vi "DAISY_PAR_HV_slow_control_2_16.vi"() -> ()   [LabVIEW 2018]
uses:
  4623b864-5764-45c6-9cb2-3e18237880ca.vi
  fa57f61f-0bb9-49ac-92eb-fcb40add4dbb.vi
  <vilib>/DAQmx/read.llb/DAQmx Read (Analog 1D DBL NChan 1Samp).vi
  ffb0d1b3-ef19-4e2e-b36e-7277177ef4b3.vi
  9a1acc8a-69db-4048-9e4c-bb07d66d2422.vi
  <vilib>/DAQmx/create/channels.llb/DAQmx Create Channel (AI-Voltage-Basic).vi
  <vilib>/DAQmx/create/channels.llb/DAQmx Create Channel (AI-Current-Basic).vi
  <vilib>/DAQmx/create/channels.llb/DAQmx Create Channel (AI-Temperature-RTD).vi
  <vilib>/DAQmx/miscellaneous.llb/DAQmx Fill In Error Info.vi
  <vilib>/Utility/file.llb/Read Delimited Spreadsheet (string).vi
  <instrlib>/Lake Shore 335/Lake Shore 335.lvlib
  <instrlib>/CAEN PSM/CAEN PSM.lvlib
  <resource>/objmgr/daqmx.rc
panel:
  out "Setpoint (°C)":dbl
  out "Heater Range":i32
  out "Heater (°C)":dbl
  out "Coldhead (°C)":dbl
  out "Cycle number":i32
  out "Alarm state":bool
  out "Timestamp last \nmeasured (UPS)":timestamp
  out "Auto-clear":bool
  in  "Auto-clear data?":bool
  in  "Clear data":bool
  in  "Clear data every N cycles":dbl=1000000.0
  in  "N samples":i32=30
  out "Average Flow (SLPM)":dbl caption="Flow (SLPM)"
  out "CAEN Ch. Names":string[](array[string])
  in  "Cycles to execute":dbl=5.0 format="%#_13g"
  out "Detector Pressure":dbl
  in  "N samples":i32=20
  in  "Allows tabs on \nfront panel":T1(tab)
  in  "Anode ch.":enum16{"1", "2", "3", "4"}(ring)=enum."3"
  in  "CAEN unit selector":enum16{"CAEN 1", "CAEN 2"}(ring)
  in  "Multipliers":dbl[](array[numeric])=[1.0, 1.0, 1.0, 1.0, 1.0, 1.0, 1.0, 1.0]
  in  "Offsets\nsubtracted":dbl[](array[numeric])=[0.0, 0.0, 0.0, 0.0, 0.0, 0.0, 0.0, 0.0]
  in  "Channel Names (9207, ai8:15)":string[](array[string])=["i0", "i1", "i2", "i3", "i4", "i5", "i6", "i7"] caption="\"Other\""
  in  "Flow meter input:":u16(ring)=3 items=["v0", "v1", "v2", "v3", "v4", "v5", "v6", "v7"]
  in  "Detector pressure input:":u16(ring) items=["v0", "v1", "v2", "v3", "v4", "v5", "v6", "v7"]
  in  "Channel Names (9207, ai0:7)":string[](array[string])=["v0", "v1", "v2", "v3", "v4", "v5", "v6", "v7"] caption="\"Other\""
  in  "Multipliers":dbl[](array[numeric])=[1.0, 1.0, 1.0, 1.0, 1.0, 1.0, 1.0, 1.0]
  in  "Offsets\nsubtracted":dbl[](array[numeric])=[0.0, 0.0, 0.0, 0.0, 0.0, 0.0, 0.0, 0.0]
  in  "Voltage channels":tag[](array[tag])=["9207/ai0", "9207/ai1", "9207/ai2", "9207/ai3", "9207/ai4", "9207/ai5", "9207/ai6", "9207/ai7"]
  in  "COM-port CAEN":refnum<visa-resource-name>
  in  "ID Query":bool
  in  "COM-port LakeShore":refnum<visa-resource-name>
  in  "PID settings":cluster{"P":dbl, "I":dbl, "D":dbl}={"P"=50.0, "I"=20.0, "D"=120.0}
  in  "Current channels":tag[](array[tag])=["9207/ai8", "9207/ai9", "9207/ai10", "9207/ai11", "9207/ai12", "9207/ai13", "9207/ai14", "9207/ai15"]
  in  "Channel Names (CAEN)":string[](array[string])=["PMT 1", "PMT 2", "Anode", "Cathode", "Top gate", "Bottom gate", "Other 1", "Other 2"]
  in  "RTD Type":i32(ring)=10071 items=["Pt3750"=12481, "Pt3851"=10071, "Pt3911"=12482, "Pt3916"=10069, "Pt3920"=10053, "Pt3928"=12483, "Custom"=10137]
  in  "Module 1 channels (slot 1)":tag[](array[tag])=["cDAQ2Mod2/ai0", "cDAQ2Mod2/ai1", "cDAQ2Mod2/ai2", "cDAQ2Mod2/ai3", "cDAQ2Mod2/ai4", "cDAQ2Mod2/ai5", "cDAQ2Mod2/ai6", "cDAQ2Mod2/ai7"]
  in  "Resistance Configuration":i32(ring)=3 items=["3-Wire"=3, "4-Wire"=4]
  in  "R (T = 0°C):":dbl=100.0 format="%_4g"
  in  "B":dbl
  in  "A":dbl
  in  "C":dbl
  in  "Module 2 channels (slot 2)":tag[](array[tag])=["cDAQ2Mod3/ai0", "cDAQ2Mod3/ai1", "cDAQ2Mod3/ai2", "cDAQ2Mod3/ai3", "cDAQ2Mod3/ai4", "cDAQ2Mod3/ai5", "cDAQ2Mod3/ai6", "cDAQ2Mod3/ai7"]
  in  "Shut off heater \nif Alarm is active":bool=TRUE
  in  "Re-save headers":bool
  in  "Resistance Configuration":i32(ring)=3 items=["3-Wire"=3, "4-Wire"=4]
  in  "Module 3 channels":tag[](array[tag])
  in  "RTD Type":i32(ring)=12481 items=["Pt3750"=12481, "Pt3851"=10071, "Pt3911"=12482, "Pt3916"=10069, "Pt3920"=10053, "Pt3928"=12483, "Custom"=10137]
  in  "R (T = 0°C)":dbl=1000.0 format="%0.1f"
  in  "Ignore Initialization Errors":bool=TRUE caption="Ignore init. errors?"
  out "Started up?":bool
  in  "9216 Timing Mode":i32(ring)=14712 items=["High Resolution"=10195, "High Speed"=14712]
  in  "9207 Timing Mode":i32(ring)=14712 items=["High Resolution"=10195, "High Speed"=14712]
  in  "9226 Timing Mode":i32(ring)=14712 items=["High Resolution"=10195, "High Speed"=14712]
  in  "Kill all channels (Trip)":bool
  in  "Scale.Range:Minimum 8":dbl
  in  "Scale.Range:Maximum 8":dbl=4000.0
  in  "Scale.Range:Minimum 7":dbl
  in  "Scale.Range:Maximum 7":dbl=4000.0
  in  "Scale.Range:Minimum 6":dbl=-3000.0
  in  "Scale.Range:Maximum 6":dbl
  in  "Scale.Range:Minimum 5":dbl
  in  "Scale.Range:Maximum 5":dbl=3000.0
  in  "Scale.Range:Minimum 4":dbl=-5000.0
  in  "Scale.Range:Maximum 4":dbl
  in  "Scale.Range:Maximum 3":dbl=4000.0
  in  "Scale.Range:Minimum 3":dbl
  in  "Scale.Range:Maximum 2":dbl=1000.0
  in  "Scale.Range:Minimum 2":dbl
  out "CAEN 1.1":dbl(knob) scale=0.0..1000.0
  out "CAEN 1.1":string
  in  "Scale.Range:Maximum":dbl=1000.0
  in  "Scale.Range:Minimum":dbl
  out "CAEN 2.3 2":string
  out "CAEN 2.2 2":string
  out "Channel Names":string[](array[string])
  out "CAEN 2.3":dbl(knob) scale=0.0..4000.0
  out "CAEN 2.2":dbl(knob) scale=0.0..4000.0
  out "CAEN 2.1":string
  out "CAEN 2.0":string
  out "CAEN 1.3":string
  out "CAEN 1.2":string
  out "CAEN 1.0":string
  out "Channel Names":string[](array[string])
  in  "Set to zero (ramp down)":bool
  out "CAEN 2.1":dbl(knob) scale=0.0..-3000.0
  out "CAEN 2.0":dbl(knob) scale=0.0..3000.0
  in  "Apply Voltage":bool
  in  "VSet (V)":dbl[](array[numeric])
  in  "IMax (uA)":sgl[](array[numeric])
  in  "VMax (V)":u16[](array[numeric])
  out "CAEN 1.3":dbl(knob) scale=0.0..-5000.0
  out "CAEN 1.2":dbl(knob) scale=0.0..4000.0
  out "CAEN 1.0":dbl(knob) scale=0.0..1000.0
  out "Vmon (V)":dbl[](array[numeric])
  out "IMon (uA)":dbl[](array[numeric])
  in  "Reset anode\nperiodically?":bool
  in  "Kill every Y minutes":i32=10
  in  "Keep off for X seconds":i32=10
  out "?":bool
  out "Killed":bool
  out "Restarted":bool
  out "Anode timers":timestamp[](array[timestamp])
  out "Seconds until \nanode autokill":dbl format="%.2g"
  out "Seconds until \nanode reset":dbl format="%.2g"
  in  "Temperature channel selector":u16(ring) items=["0"=0, "1"=1, "2"=2, "3"=3, "4"=4, "5"=5, "6"=6, "7"=7, "Average"=666]
  out "Heater power (%)":cluster{timestamp[], dbl[]}[](graph)
  out "Flow (SLPM)":cluster{timestamp[], dbl[]}[](graph)
  out "9207 (ai 0:7, Volts)":cluster{timestamp[], dbl[]}[](graph)
  out "Phase Diagram":cluster{"X":dbl, "Y":dbl}[](graph)
  out "Setup Temperature (9216 0:15, °C)":cluster{timestamp[], dbl[]}[](graph)
  out "LakeShore readings":dbl[](array[numeric])
  out "Low Temperature (9226 0:7 and LakeShore A;B, °C)":cluster{timestamp[], dbl[]}[](graph)
  in  "Reset?":bool
  out "Integrated Flow (SL)":dbl
  in  "Pause?":bool
  in  "Setpoint (°C)":dbl=-100.0 format="%.1f"
  in  "Heater range":u16(ring) items=["Off", "Low (On)", "Medium", "High"]
  in  "\"Sound\" alarm":bool
  in  "Sound alarm\nFrequency (Hz)":dbl=1260.0
  in  "Send status email now":bool
  out "Email error":i32
  out "source":string
  in  "Number of Bonus lines":i32=1
  out "Names (optional)":string[](array[string])
  in  "Send daily email?":bool=TRUE
  in  "Phone numbers":string[](array[string])
  out "Alarm (or test) message":string
  in  "Alarm\nMaster switch":bool
  in  "Repeat Alarm SMS\nevery N minutes":dbl=15.0
  in  "Test alarm":bool
  out "Warning":bool
  in  "UPS":bool
  in  "UPS Voltage \nLower Threshold":dbl=220.0
  out "NI mod 2&3 status":bool
  in  "NI mod 2&3":bool
  in  "NI mod 1":bool
  in  "CAEN 2":bool
  in  "CAEN 1":bool
  in  "LakeShore":bool
  out "Det. P. warning":bool
  out "Boolean 6":bool
  out "Boolean 5":bool
  out "Boolean 4":bool
  out "Boolean 3":bool
  out "Boolean 2":bool
  out "Boolean":bool
  in  "T 6":bool
  in  "T 5":bool
  in  "T 4":bool
  in  "T 3":bool
  in  "T 2":bool
  in  "T 1":bool
  in  "Detector Pressure":bool
  in  "Overpressure threshold":dbl
  in  "Underpressure threshold":dbl
  out "Comm. status":bool
  in  "High Temp threshold":dbl format="%#_13g"
  in  "Low Temp threshold":dbl format="%#_13g"
  out "LakeShore status":bool
  out "NI mod1 (P) status":bool
  out "CAEN 1 status":bool
  out "CAEN 2 status":bool
  out "Initialization status":bool
  out "Minimum input voltage measured":dbl
  out "Alarm active 2":bool
  out "SMS error":string
  out "Status email preview":string
  in  "Send status email at time:":string="14:00"
  in  "Email Addresses":string[](array[string])
  in  "return address":string="xamsups@gmail.com"
  out "NI 9226":errorcluster
  in  "HV Channel status":string="Click the button to request the latest High Voltage channel status.\nView another channel with the arrows, or typing 0 through 3."
  out "CAEN 1":T2(array[cluster])
  out "CAEN 2":T2(array[cluster])
  in  "Query HV status":bool
  in  "LabVIEW error code":string="Google this"
  in  "String 7":string="A checkmark means \"No error\" and false. A red X means an error occurred"
  out "\"status\"":bool
  in  "\"source\"":string="This may show two things: the latest executed VI in the task chain, in reverse order, or: which VI produced an error, with a short description. If the error can't easily be resolved, google the code."
  out "NI 9216 x2":errorcluster
  out "CAEN 1":errorcluster
  out "CAEN 2":errorcluster
  out "Lakeshore":errorcluster
  out "NI 9207":errorcluster
  out "Temp A":dbl
  out "Temp B":dbl
  in  "Temperature Channel Selector":u16(ring) items=["0", "1", "2", "3", "4", "5", "6", "7"]
  out "Historical Large Phase Diagram":cluster{dbl[], dbl[]}[](graph)
  out "Large Phase Diagram":cluster{"X":dbl, "Y":dbl}[](graph)
  in  "Temperature Channel Selector":u16(ring) items=["0"=0, "1"=1, "2"=2, "3"=3, "4"=4, "5"=5, "6"=6, "7"=7, "Average"=666]
  out "PT1000 data":dbl[](array[numeric]) format="%0.2f"
  out "9207 (V; A) Converted":dbl[](array[numeric])
  out "9216 #1 (°C)":dbl[](array[numeric])
  out "9216 #2 (°C)":dbl[](array[numeric])
  out "Raw readouts (V, mA)":dbl[](array[numeric]) format="%0.2f"
  out "Det.P input #":i32
  out "Flow input #":i32
  out "PT100 data":dbl[](array[numeric]) format="%0.2f"
  out "Polarity signs":dbl[](array[numeric])
  out "9207 (ai 8:15, Amperes)":cluster{timestamp[], dbl[]}[](graph)
  in  "Kill voltage":bool
  in  "stop":bool
  out "Voltages":dbl[](array[numeric])
  out "Time until next cycle":dbl format="%.3g"
  in  "Time per cycle (s)":i32=2 caption="Time Target (s)"
  # "Moving Averages"
  # "CAEN settings"
  # "NI 9216 Temperature settings"
  # "NI 9207 Voltage settings"
  # "NI 9207 Current settings"
  # "If RTD type is custom,\nspecify the Callendar-\nVan Dusen parameters"
  # "Anode connected to:"
  # "Channel:"
  # "Lakeshore settings"
  # "NI 9226 Temperature settings"
  # "Miscellaneous"
  # "Gain (P) (XX.X)"
  # "Reset (I) (XX.X)"
  # "Rate (D) (X.X%)"
  # "Data"
  # "Scale:"
  # "to"
  # "to"
  # "Scale:"
  # "Time of last reset"
  # "Time of last reactivation"
  # "to"
  # "Scale:"
  # "to"
  # "Scale:"
  # "Settings"
  # "Scale:"
  # "to"
  # "Scale:"
  # "to"
  # "Scale:"
  # "to"
  # "to"
  # "Scale:"
  # "Alarm indicators and arms"
  # "Detector Thresholds"
  # "Daily status email"
  # "SMS and sound alarm"
  # "Alarm conditions"
  # "Temperature channels:"
  # "Uninterruptable Power Supply"
  # "Task/error information"
  # "High Voltage channel status"
  # "Error info example"
  # "Channel"
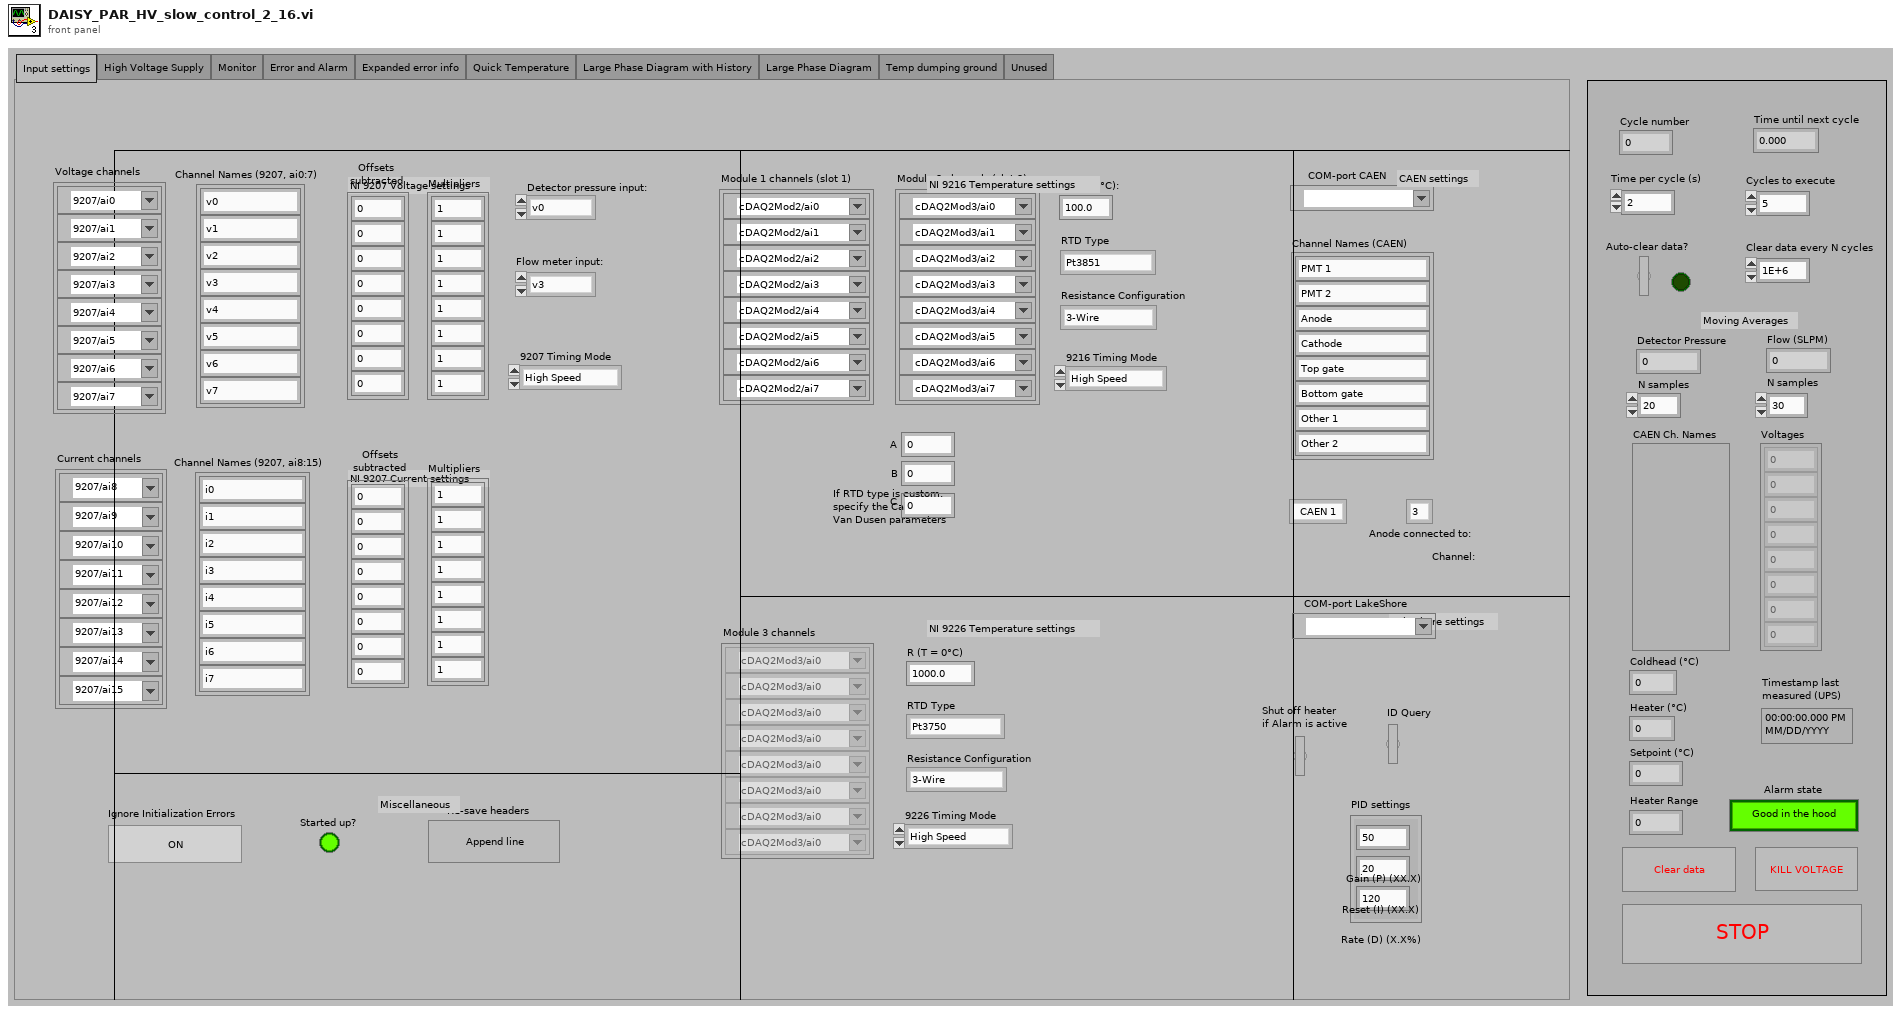
[diagram p1: front panel]
types:
  T1 = enum32{"Input settings", "High Voltage Supply", "Monitor", "Error and Alarm", "Expanded error info", "Quick Temperature", "Large Phase Diagram with History", "Large Phase Diagram", "Temp dumping ground", "Unused"}
  T2 = cluster{"ON":bool, "RUP":bool, "RDW":bool, "OVC":bool, "OVV":bool, "UNV":bool, "MAXV":bool, "TRIP":bool, "OVP":bool, "OVT":bool, "DIS":bool, "KILL":bool, "ILK":bool, "NOCAL":bool}[]
  T3 = cluster{"Baud Rate":u32, "Parity":u16, "Data Bits":u16, "Stop Bits":u16, "Flow Control":u16}
  T4 = typedef "CAEN PSM.lvlib/BoardHandle.ctl" = cluster{"VISA resource name":refnum<visa-resource-name>, "Board address":u8, "NChannels":u8}
  T5 = cluster{"task out":refnum<k21>, "error out":errorcluster}
  T6 = cluster{"VISA resource name out":refnum<visa-resource-name>, "error out":errorcluster}
  T7 = cluster{"VISA resource name":refnum<visa-resource-name>, "Board address":u8, "NChannels":u8}[]
  T8 = cluster{"VISA resource name":refnum<visa-resource-name>, "Board address":u8, "NChannels":u8}
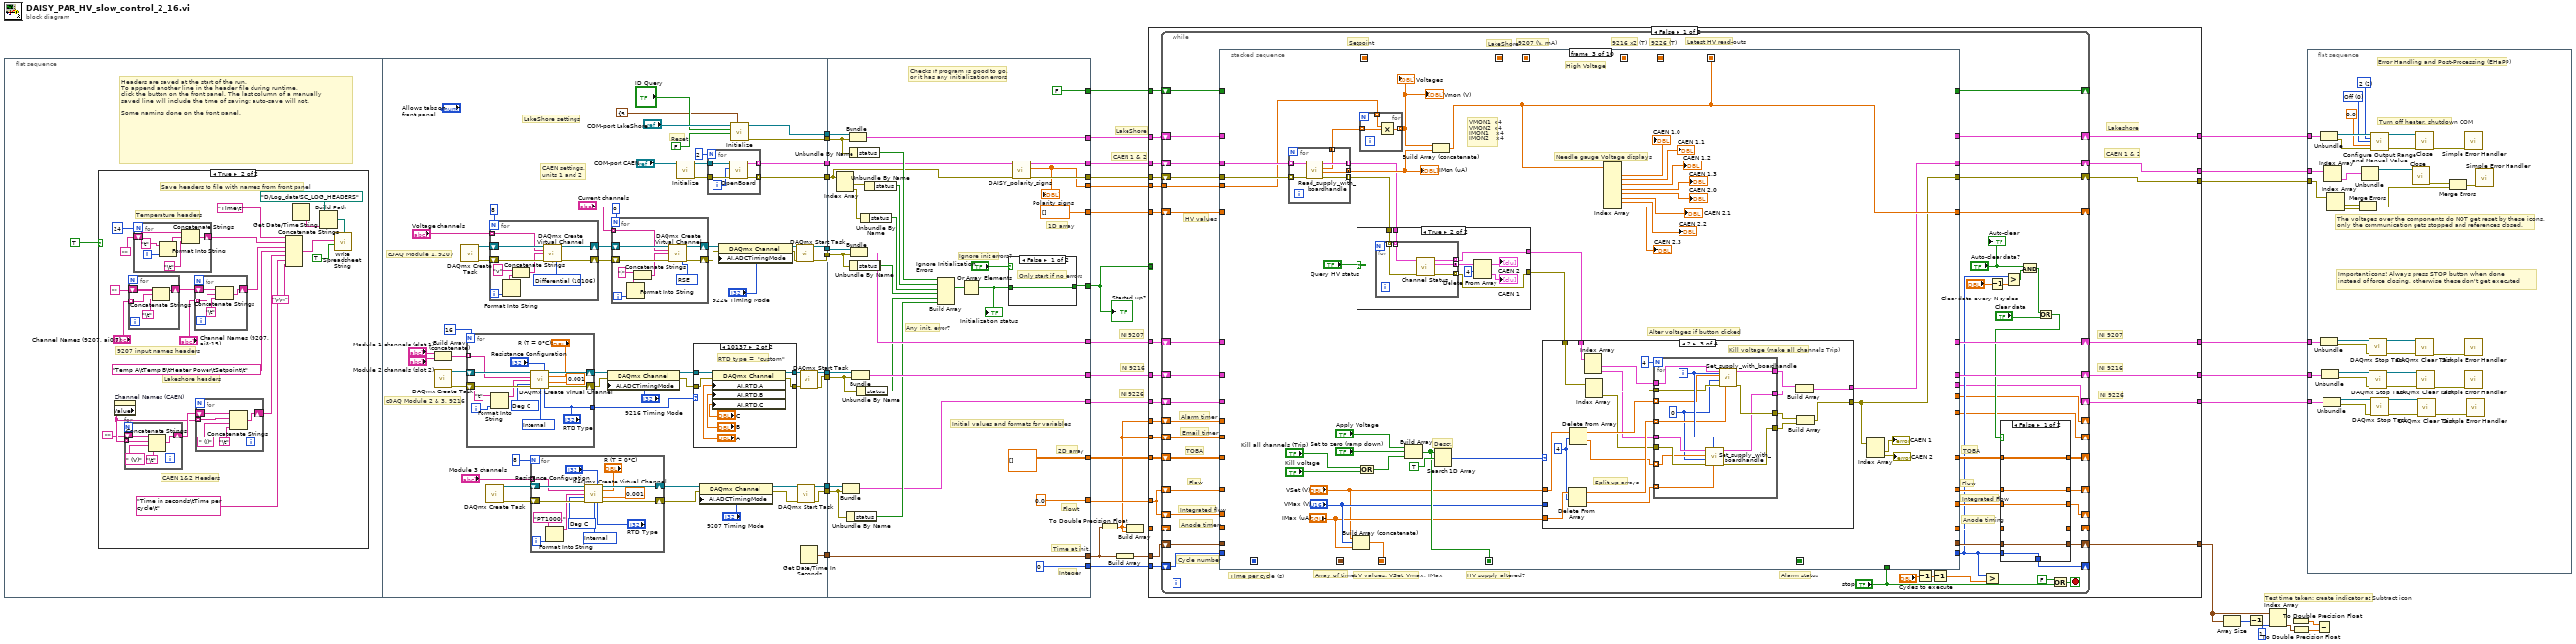
[diagram p0: block diagram]
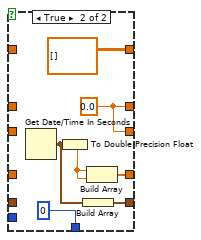
[diagram p2: hidden frame]
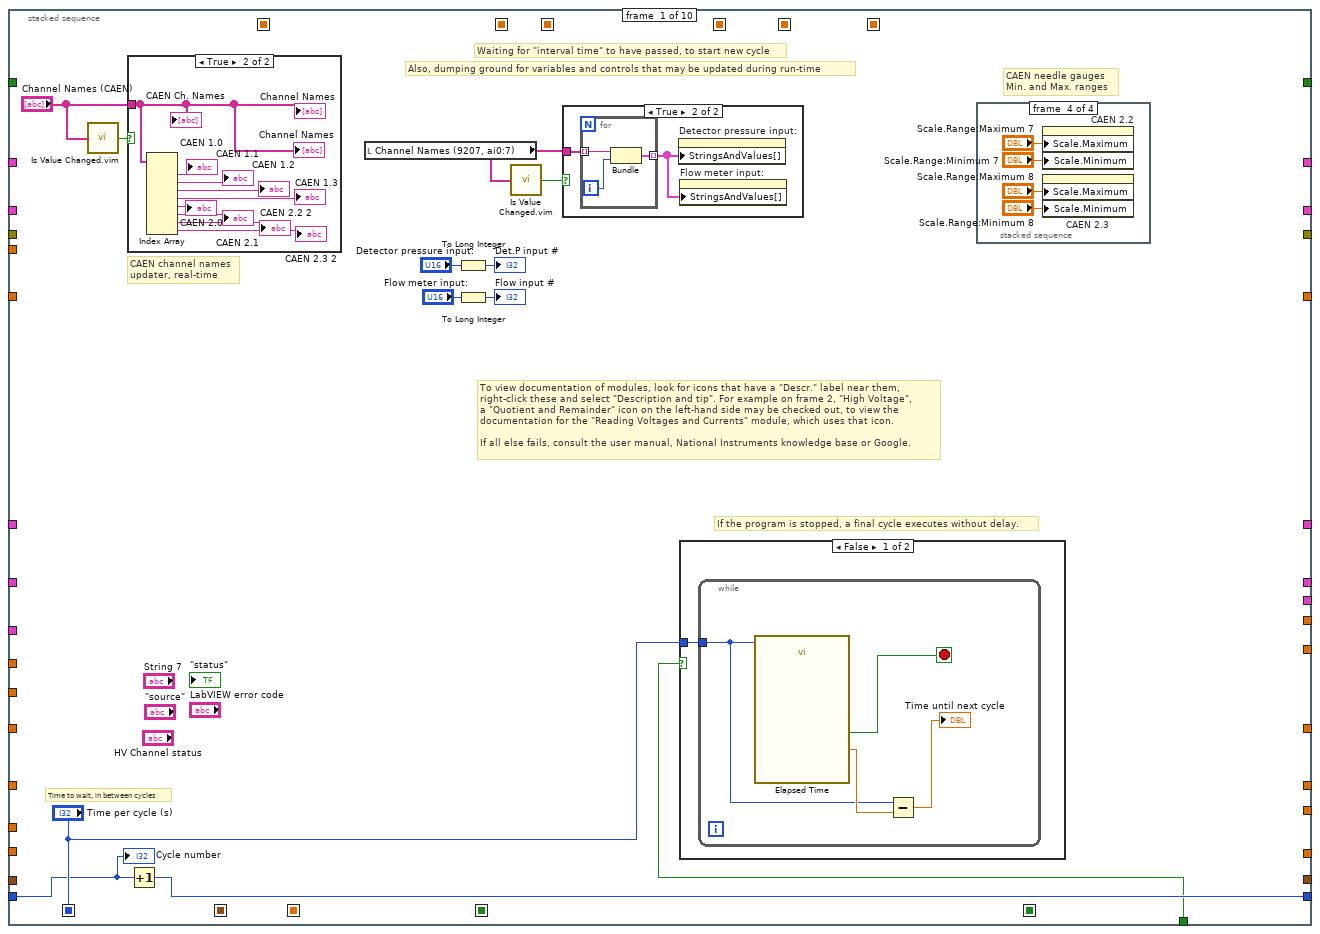
[diagram p3: hidden frame]
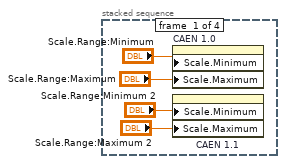
[diagram p6: hidden frame]
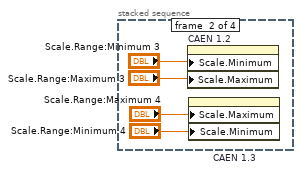
[diagram p7: hidden frame]
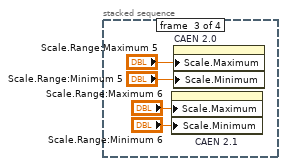
[diagram p8: hidden frame]
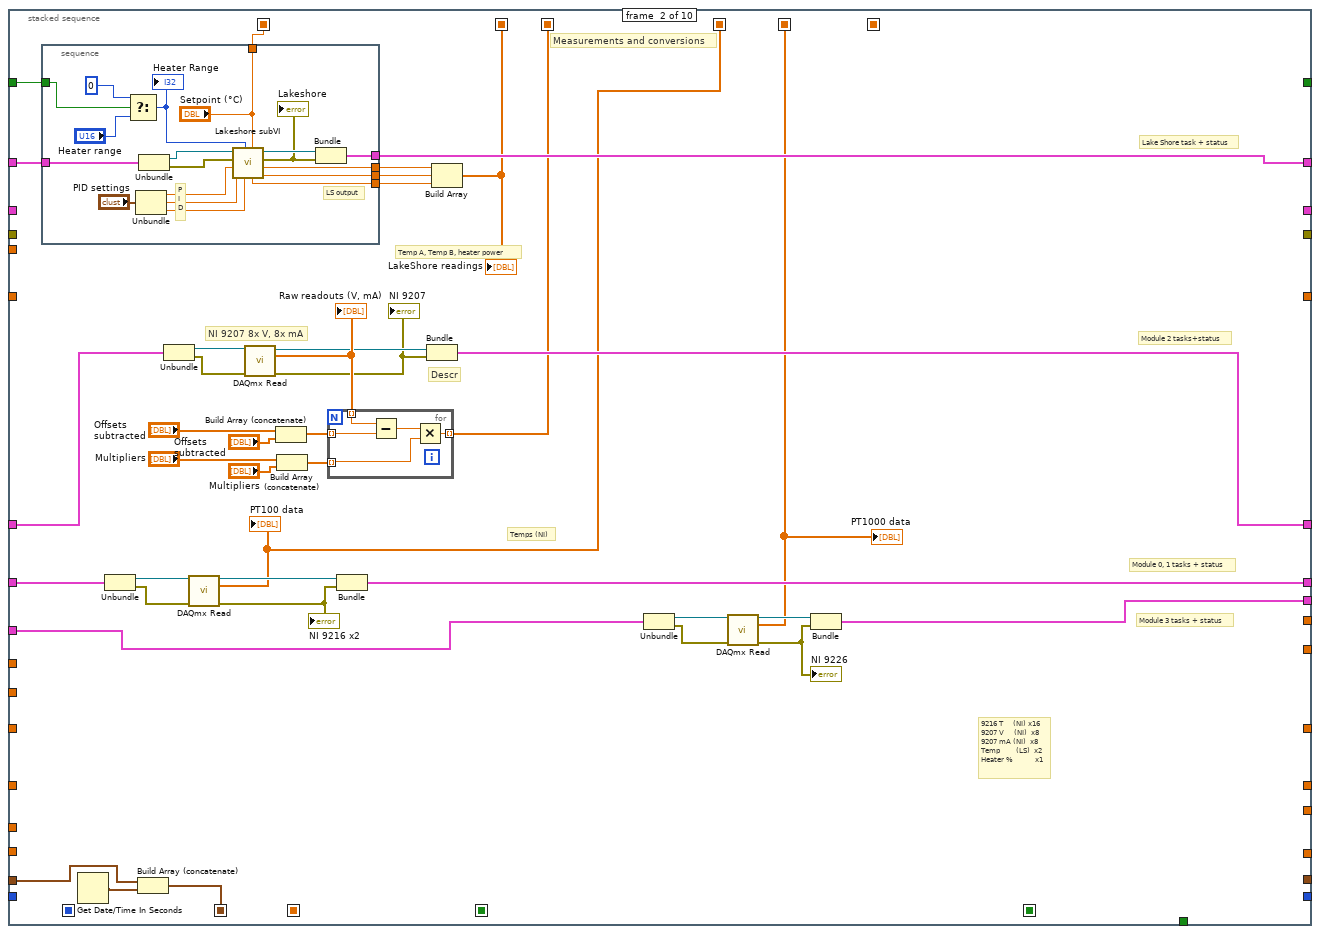
[diagram p10: hidden frame]
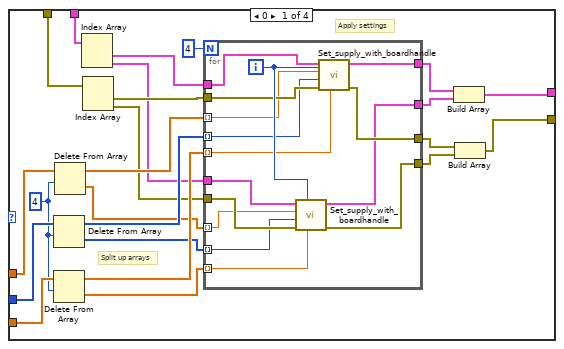
[diagram p11: hidden frame]
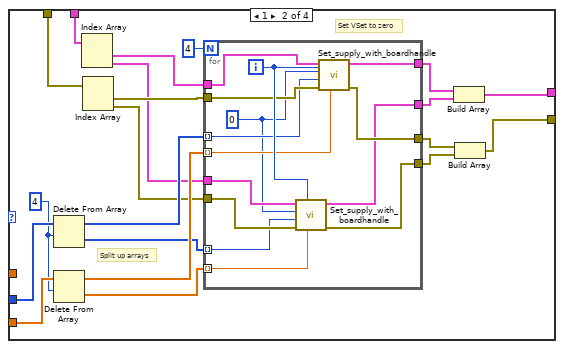
[diagram p12: hidden frame]
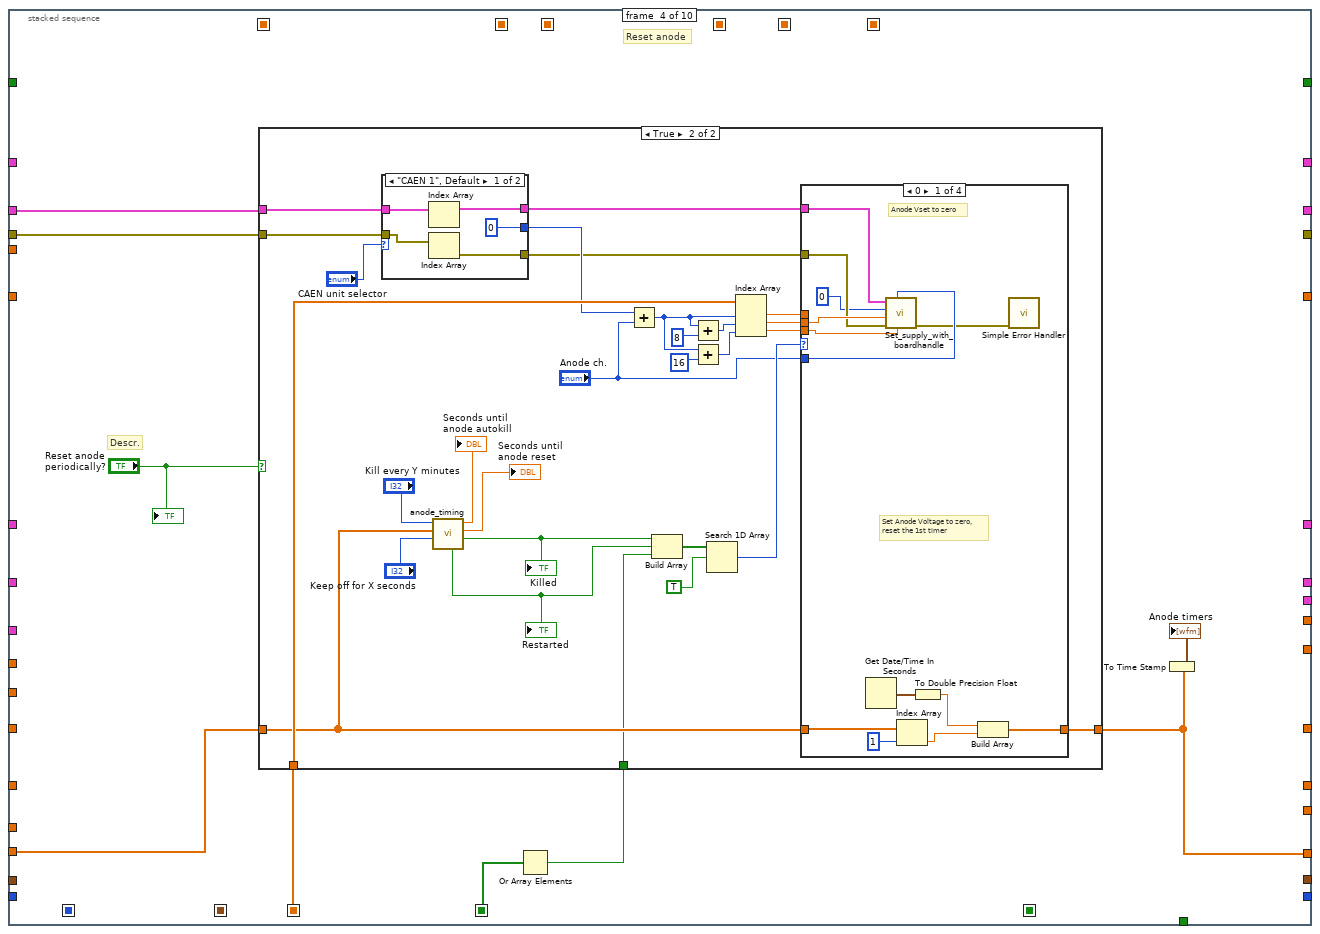
[diagram p15: hidden frame]
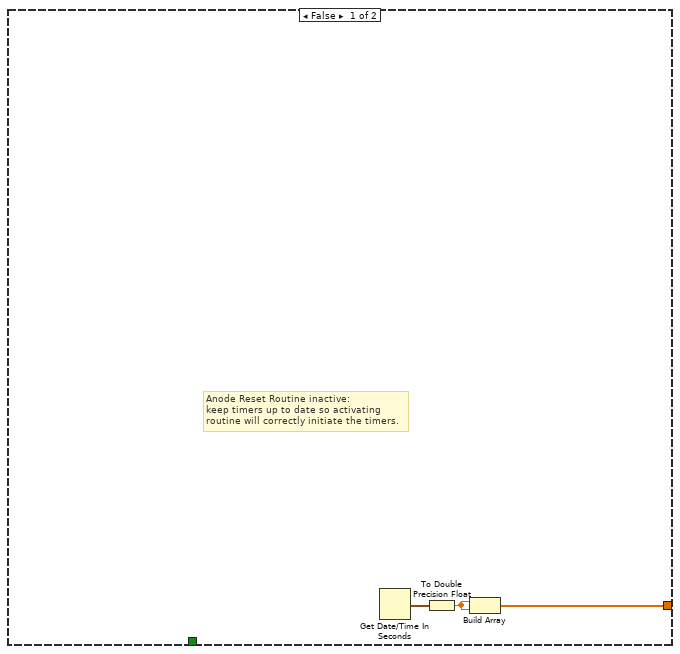
[diagram p16: hidden frame]
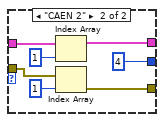
[diagram p17: hidden frame]
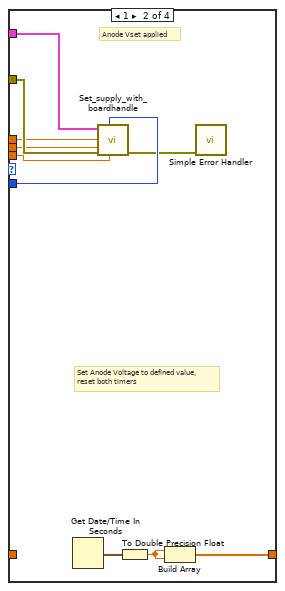
[diagram p18: hidden frame]
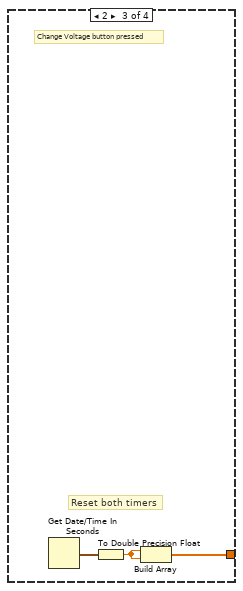
[diagram p19: hidden frame]
diagram:
  # "NI 9226"
  # "NI 9216"
  # "Test time taken: create indicator at Subtract icon"
  # "NI 9207"
  # "CAEN 1 & 2"
  # "LakeShore"
  n1 = flat-sequence {
    tunnel: [w140] -> w42
    tunnel: [w139] -> w41
    tunnel: [w136] -> w40
    tunnel: [w127] -> w39
    tunnel: [w135] -> w35
    tunnel: [w128] -> w21
    tunnel: [w122] -> w14
    tunnel: [w121] -> w13
    tunnel: [w110] -> w9
    tunnel: [w109] -> w8
    tunnel: [w106] -> w4
    tunnel: w42 -> [w237]
    tunnel: w41 -> [w236]
    tunnel: w40 -> [w208]
    tunnel: w39 -> [w229]
    tunnel: [w238] -> w27
    tunnel: [0.0] -> w26
    tunnel: [dbl[] []] -> w38
    tunnel: [dbl[][] []] -> w15
    tunnel: [0] -> w37
    tunnel: [w235] -> w36
    tunnel: [w234] -> w25
    tunnel: w35 -> [w234]
    tunnel: [FALSE] -> w22
    tunnel: w21 -> [w230]
    tunnel: [w228] -> w20
    tunnel: w14 -> [w221]
    tunnel: w13 -> [w220]
    tunnel: [w219] -> w12
    tunnel: w9 -> [w216]
    tunnel: w8 -> [w215]
    tunnel: [w213] -> w7
    tunnel: [w206] -> w5
    tunnel: w4 -> [w210]
    tunnel: [w209] -> w3
    tunnel: [w207] -> w2
    frame #0 {
      # "Headers are saved at the start of the run.\nTo append another line in the header file during runtime,\nclick the button on the front panel. The last column of a manually\nsaved line will include the time of saving; auto-save will not.\n\nSome naming done on the front panel."
      n2 = case shown="True" TRUE {
        frame False {
        }
        frame True {
          # "CAEN 1&2 Headers"
          # "Lakeshore headers"
          # "9207 input names headers"
          # "Temperature headers"
          # "Save headers to file with names from front panel"
          n3 = property on="Channel Names (CAEN)" class="Arr (strict)"() -> ("Value"=w49:string[])  [unwired: 2 in, 2 out]
          n4 = for {
            tunnel: w49 -> [w73] mode=indexing
            shift-right: [w71] -> w50
            shift-left: "" -> [w70]
            n5 = Concatenate Strings(w70, w73, " (V)", "\t") -> (w71:string)
          }
          n6 = for {
            shift-right: [w81] -> w53
            shift-left: "" -> [w82]
            tunnel: "Channel Names (9207, ai0:7)" -> [w79] mode=indexing
            n7 = Concatenate Strings(w82, w79, "\t") -> (w81:string)
          }
          n8 = for {
            N: 24 -> [_]
            shift-right: [w83] -> w56
            shift-left: "" -> [w84]
            i -> [w88]
            n9 = Format Into String(initial string="t", w88) -> (resulting string=w86:string)  [unwired: 2 in, 1 out]
            n10 = Concatenate Strings(w84, w86, "\t") -> (w83:string)
          }
          n11 = for {
            shift-right: [w76] -> w52
            shift-left: w53 -> [w78]
            tunnel: "Channel Names (9207, ai8:15)" -> [w75] mode=indexing
            n12 = Concatenate Strings(w78, w75, "\t") -> (w76:string)
          }
          n13 = for {
            shift-right: [w66] -> w48
            shift-left: w50 -> [w67]
            tunnel: w49 -> [w65] mode=indexing
            n14 = Concatenate Strings(w67, w65, " (I)", "\t") -> (w66:string)
          }
          n15 = Concatenate Strings("Time\t", w56, w52, "Temp A\tTemp B\tHeater Power\tSetpoint\t", w48, "Time in seconds\tTime per cycle\t", "\r\n") -> (w55:string)
          n16 = Get Date/Time String() -> (date string=w59:string)  [unwired: 3 in, 1 out]
          n17 = Build Path(base path=path "D:/Log_data/SC_LOG_HEADERS" ("file path (dialog if empty)"), name or relative path=w59) -> (appended path=w60:path)
          n18 = call <vilib>:"Write Spreadsheet String.vi"("append to file? (new file:F)"=TRUE, "spreadsheet string"=w55, "file path (dialog if empty)"=w60) -> ()  [unwired: 7 in, 2 out]
        }
      }
    }
    frame #1 {
      # "cDAQ Module 2 & 3, 9216"
      # "cDAQ Module 1, 9207"
      # "CAEN settings,\nunits 1 and 2"
      # "Reset"
      # "LakeShore settings"
      n19 = call <vilib>:"DAQmx Create Task.vi"() -> ("task out"=w107:refnum<k21>, "error out"=w123:errorcluster)  [unwired: 14 in]
      n20 = Build Array (concatenate)("Module 1 channels (slot 1)", "Module 2 channels (slot 2)") -> (w118:tag[])
      n21 = call <vilib>:"DAQmx Create Task.vi"() -> ("task out"=w132:refnum<k21>, "error out"=w131:errorcluster)  [unwired: 14 in]
      n22 = for {
        N: 16 -> [_]
        shift-right: [w182] -> w98
        shift-left: w107 -> [w185]
        shift-right: [w183] -> w96
        shift-left: w123 -> [w184]
        tunnel: w118 -> [w181] mode=indexing
        tunnel: ["RTD Type"] -> w115
        i -> [w179]
        w177 = 10200 items=["Internal"=10200, "External"=10167, "None"=10230] ("Current Excitation Source")
        w176 = 10143 items=["Deg C"=10143, "Deg F"=10144, "Kelvins"=10325, "Deg R"=10145, "From Custom Scale"=10065] ("units")
        n23 = Format Into String(initial string="t", w179) -> (resulting string=w178:string)  [unwired: 2 in, 1 out]
        n24 = call-poly <vilib>:"DAQmx Create Virtual Channel.vi"("task in"=w185, "resistance configuration"="Resistance Configuration", "physical channels"=w181, "r0"="R (T = 0°C):", "name to assign"=w178, "units"=w176, "current excitation value"=0.001, "error in"=w184, "current excitation source"=w177, "rtd type"="RTD Type") -> ("task out"=w182:refnum<k21>, "error out"=w183:errorcluster)  [unwired: 4 in]
      }
      n25 = call <vilib>:"DAQmx Create Task.vi"() -> ("task out"=w113:refnum<k21>, "error out"=w112:errorcluster)  [unwired: 14 in]
      n26 = for {
        N: 8 -> [_]
        shift-right: [w201] -> w104
        shift-left: w132 -> [w200]
        shift-right: [w202] -> w129
        shift-left: w131 -> [w198]
        tunnel: "Voltage channels" -> [w199] mode=indexing
        i -> [w204]
        w196 = 10106 items=["Default"=-1, "RSE"=10083, "NRSE"=10078, "Differential"=10106, "Pseudodifferential"=12529] ("input terminal configuration")
        n27 = Format Into String(w204) -> (resulting string=w203:string)  [unwired: 3 in, 1 out]
        n28 = Concatenate Strings("v" ("string"), w203) -> (w197:string)
        n29 = call-poly <vilib>:"DAQmx Create Virtual Channel.vi"("task in"=w200, "input terminal configuration"=w196, "physical channels"=w199, "name to assign"=w197, "error in"=w198) -> ("task out"=w201:refnum<k21>, "error out"=w202:errorcluster)  [unwired: 9 in]
      }
      n30 = for {
        N: 8 -> [_]
        shift-right: [w160] -> w103
        shift-left: w113 -> [w159]
        shift-right: [w161] -> w102
        shift-left: w112 -> [w162]
        tunnel: "Module 3 channels" -> [w157] mode=indexing
        i -> [w155]
        w151 = 10200 items=["Internal"=10200, "External"=10167, "None"=10230] ("current excitation source")
        w153 = 10143 items=["Deg C"=10143, "Deg F"=10144, "Kelvins"=10325, "Deg R"=10145, "From Custom Scale"=10065] ("units")
        n31 = Format Into String(initial string="PT1000.", w155) -> (resulting string=w154:string)  [unwired: 2 in, 1 out]
        n32 = call-poly <vilib>:"DAQmx Create Virtual Channel.vi"("task in"=w159, "resistance configuration"="Resistance Configuration", "physical channels"=w157, "r0"="R (T = 0°C)", "name to assign"=w154, "units"=w153, "current excitation value"=0.001, "error in"=w162, "current excitation source"=w151, "rtd type"="RTD Type") -> ("task out"=w160:refnum<k21>, "error out"=w161:errorcluster)  [unwired: 4 in]
      }
      n33 = property class="DAQmx Channel"(reference=w98, error in=w96, "AI.ADCTimingMode"="9216 Timing Mode") -> (reference out=w97:refnum<k21>, error out=w95:errorcluster)
      n34 = for {
        N: 8 -> [_]
        shift-right: [w187] -> w93
        shift-left: w104 -> [w194]
        shift-right: [w186] -> w90
        shift-left: w129 -> [w193]
        tunnel: "Current channels" -> [w192] mode=indexing
        i -> [w191]
        w195 = 10083 items=["default"=-1, "RSE"=10083, "NRSE"=10078, "Differential"=10106, "Pseudodifferential"=12529] ("input terminal configuration")
        n35 = Format Into String(w191) -> (resulting string=w189:string)  [unwired: 3 in, 1 out]
        n36 = Concatenate Strings("i", w189) -> (w188:string)
        n37 = call-poly <vilib>:"DAQmx Create Virtual Channel.vi"("task in"=w194, "input terminal configuration"=w195, "physical channels"=w192, "name to assign"=w188, "error in"=w193) -> ("task out"=w187:refnum<k21>, "error out"=w186:errorcluster)  [unwired: 9 in]
      }
      n38 = call <instrlib>:"Initialize.vi"("VISA resource name"="COM-port CAEN") -> ("error out"=w137:errorcluster, "VISA resource name out"=w133:refnum<visa-resource-name>)  [unwired: 9 in]
      n39 = case shown="10137" w115 {
        tunnel: w97 -> [w164 w168]
        tunnel: w95 -> [w163 w167]
        tunnel: [w164 w166] -> w117
        tunnel: [w163 w165] -> w116
        frame 0, Default {
          # "Don't need to specify the A, B, C\nvalues if RTD type is not \"custom\""
        }
        frame 10137 {
          # "RTD type =  \"custom\""
          n40 = property class="DAQmx Channel"(reference=w168, error in=w167, "AI.RTD.A"="A", "AI.RTD.B"="B", "AI.RTD.C"="C") -> (reference out=w166:refnum<k21>, error out=w165:errorcluster)
        }
      }
      n41 = property class="DAQmx Channel"(reference=w103, error in=w102, "AI.ADCTimingMode"="9207 Timing Mode") -> (reference out=w100:refnum<k21>, error out=w99:errorcluster)
      n42 = for {
        N: 2 -> [_]
        tunnel: w133 -> [w146]
        tunnel: [w144] -> w106 mode=indexing
        tunnel: w137 -> [w148]
        tunnel: [w147] -> w136 mode=indexing
        i -> [w145]
        n43 = call <instrlib>:"OpenBoard.vi"("error in (no error)"=w148, "Board Address"=w145, "VISA resource name"=w146) -> ("error out"=w147:errorcluster, "BoardHandle"=w144:T4)  [unwired: 7 in]
      }
      n44 = property class="DAQmx Channel"(reference=w93, error in=w90, "AI.ADCTimingMode"="9226 Timing Mode") -> (reference out=w92:refnum<k21>, error out=w91:errorcluster)
      n45 = call <instrlib>:"Initialize.vi"("Serial Configuration"=T3 {"Baud Rate"=57600, "Parity"=1, "Data Bits"=7, "Stop Bits"=10, "Flow Control"=0}, "Reset (True)"=FALSE ("Reset (LakeShore)"), "ID Query (True)"="ID Query", "VISA resource name"="COM-port LakeShore") -> ("error out"=w139:errorcluster, "VISA resource name out"=w140:refnum<visa-resource-name>)  [unwired: 6 in]
      n46 = call <vilib>:"DAQmx Start Task.vi"("task/channels in"=w92, "error in"=w91) -> ("task out"=w128:refnum<k21>, "error out"=w127:errorcluster)  [unwired: 12 in]
      n47 = call <vilib>:"DAQmx Start Task.vi"("task/channels in"=w100, "error in"=w99) -> ("task out"=w110:refnum<k21>, "error out"=w109:errorcluster)  [unwired: 12 in]
      n48 = call <vilib>:"DAQmx Start Task.vi"("task/channels in"=w117, "error in"=w116) -> ("task out"=w122:refnum<k21>, "error out"=w121:errorcluster)  [unwired: 12 in]
      n49 = Get Date/Time In Seconds() -> (seconds since 1Jan1904=w135:timestamp)
    }
    frame #2 {
      # "1D array"
      # "Initial values and formats for variables"
      # "Time at init."
      # "Integer"
      # "2D array"
      # "Flowt"
      # "Checks if program is good to go,\nor it has any initialization errors"
      # "Ignore init errors?"
      # "Any init. error?"
      n50 = Index Array(array=w208) -> (element #1=w212:errorcluster, element #2=w211:errorcluster)  [unwired: 2 in]
      n51 = Bundle("task out"=w216, "error out"=w215) -> (w213:T5)  [unwired: 1 in]
      n52 = Unbundle By Name(w215) -> ("status"=w214:bool)
      n53 = Unbundle By Name(w236) -> ("status"=w222:bool)
      n54 = Bundle("VISA resource name out"=w237, "error out"=w236) -> (w235:T6)  [unwired: 1 in]
      n55 = Unbundle By Name(w229) -> ("status"=w223:bool)
      n56 = Bundle("task out"=w230, "error out"=w229) -> (w228:T5)  [unwired: 1 in]
      n57 = Bundle("task out"=w221, "error out"=w220) -> (w219:T5)  [unwired: 1 in]
      n58 = Unbundle By Name(w220) -> ("status"=w218:bool)
      n59 = Unbundle By Name(w211) -> ("status"=w233:bool)
      n60 = Unbundle By Name(w212) -> ("status"=w239:bool)
      n61 = Build Array(w222, w239, w223, w233, w218, w214) -> (w240:bool[])
      n62 = Or Array Elements(Boolean array=w240) -> (logical OR=w217:bool)
      "Initialization status" <- w217
      n63 = case shown="False" "Ignore Initialization Errors" {
        tunnel: [w241 FALSE] -> w238
        tunnel: w217 -> [w241 _]
        frame False {
          # "Only start if no errors"
        }
        frame True {
          # "Always start program"
        }
      }
      n64 = call "DAISY_polarity_signs.vi"("Errors in"=w208, "BoardHandles"=w210) -> ("Errors out"=w207:errorcluster[], "Polarity signs"=w206:dbl[], "BoardHandles Out"=w209:T7)  [unwired: 7 in]
      "Polarity signs" <- w206
    }
  }
  n65 = To Double Precision Float(number=w25) -> (double precision float=w10:dbl)
  n66 = Build Array(w25) -> (w34:timestamp[])
  n67 = Build Array(w10, w10) -> (w24:dbl[])
  n68 = case shown="False" w27 {
    selector: w27 -> [_ w1126]
    tunnel: [_ w1126] -> _
    tunnel: w38 -> [w260 _]
    tunnel: w37 -> [w265 _]
    tunnel: w15 -> [w264 _]
    tunnel: w36 -> [w261 w1124]
    tunnel: w34 -> [w263 _]
    tunnel: [w262 timestamp[] []] -> w30
    tunnel: w26 -> [w256 _]
    tunnel: w24 -> [w259 _]
    tunnel: [w258 w1124] -> w23
    tunnel: w22 -> [w257 _]
    tunnel: w20 -> [w255 w1123]
    tunnel: [w254 w1120] -> w19
    tunnel: [w253 w1123] -> w18
    tunnel: w12 -> [w252 w1122]
    tunnel: [w251 w1122] -> w11
    tunnel: w10 -> [w250 _]
    tunnel: w10 -> [w249 _]
    tunnel: w7 -> [w248 w1121]
    tunnel: [w247 w1121] -> w6
    tunnel: w5 -> [w246 _]
    tunnel: w3 -> [w245 w1120]
    tunnel: w2 -> [w244 w1119]
    tunnel: [w243 w1119] -> w1
    frame False {
      # "NI 9226"
      # "NI 9216"
      # "NI 9207"
      # "CAEN 1 & 2"
      # "Lakeshore"
      n69 = while {
        shift-right: [w281] -> _
        shift-left: w265 -> [w317]
        shift-right: [w294] -> _
        shift-left: w264 -> [w308]
        shift-right: [w286] -> w262
        shift-left: w263 -> [w314]
        shift-right: [w309] -> w254
        shift-left: w245 -> [w303]
        shift-right: [w311] -> _
        shift-left: w260 -> [w313]
        shift-right: [w310] -> w258
        shift-left: w261 -> [w312]
        shift-right: [w290] -> _
        shift-left: w256 -> [w305]
        shift-right: [w292] -> _
        shift-left: w256 -> [w306]
        shift-right: [w288] -> _
        shift-left: w259 -> [w304]
        shift-right: [w276] -> _
        shift-left: w257 -> [w302]
        shift-right: [w300] -> w253
        shift-left: w255 -> [w301]
        shift-right: [w298] -> w251
        shift-left: w252 -> [w299]
        shift-right: [w274] -> _
        shift-left: w250 -> [w275]
        shift-right: [w271] -> _
        shift-left: w249 -> [w272]
        shift-right: [w269] -> w247
        shift-left: w248 -> [w270]
        tunnel: w246 -> [w268]
        shift-right: [w266] -> w243
        shift-left: w244 -> [w267]
        stop <- w315 stop-if-true
        # "9226 (T)"
        # "Email timer"
        # "Alarm timer"
        # "Alarm status"
        # "LakeShore"
        # "9216 x2 (T)"
        # "9207 (V, mA)"
        # "HV supply altered?"
        # "Setpoint"
        # "Anode timing"
        # "Anode timers"
        # "Integrated flow"
        # "Flow"
        # "Flow"
        # "Integrated Flow"
        # "TOBA"
        # "Array of times"
        # "Latest HV read-outs"
        # "Time per cycle (s)"
        # "Cycle number"
        # "HV values: VSet, Vmax, IMax"
        # "HV values"
        # "TOBA"
        n70 = stacked-sequence {
          seq-local: [_ _ w469 _ _ _ _ _ _ _] -> [_ _ _ w614 _ _ _ _ _ _]
          seq-local: ["Time per cycle (s)" _ _ _ _ _ _ _ _ _] -> [_ _ _ _ _ _ w825 _ _ _]
          seq-local: [_ _ w453 _ _ _ _ _ _ _] -> [_ _ _ _ _ _ w823 _ _ _]
          seq-local: [_ w413 _ _ _ _ _ _ _ _] -> [_ _ _ _ w687 w808 _ _ _ _]
          seq-local: [_ _ w465 _ _ _ _ _ _ _] -> [_ _ _ w610 _ _ _ _ _ _]
          seq-local: [_ w407 _ _ _ _ _ _ _ _] -> [_ _ _ _ _ w797 w822 _ _ _]
          seq-local: [_ w405 _ _ _ _ _ _ _ _] -> [_ _ _ _ w709 w800 w820 w932 w962 w1048]
          seq-local: [_ w378 _ _ _ _ _ _ _ _] -> [_ _ _ _ w712 w803 w827 _ _ _]
          seq-local: [_ w393 _ _ _ _ _ _ _ _] -> [_ _ _ _ w711 w802 w821 _ _ _]
          seq-local: [_ _ _ _ _ _ _ w892 _ _] -> [_ _ _ _ _ _ _ _ w964 w1049]
          seq-local: [_ w381 _ _ _ _ _ _ _ _] -> [_ _ _ _ w698 w796 w819 w890 w958 w1031]
          tunnel: [w342 _ _ _ _ _ _ _ _ _] -> w280
          tunnel: "stop" -> [w341 _ _ _ _ _ _ _ _ _]
          tunnel: w317 -> [w331 _ _ _ _ _ _ _ _ _]
          tunnel: w308 -> [_ _ _ _ w741 _ _ _ _ _]
          tunnel: [_ _ _ _ w696 _ _ _ _ _] -> w295
          tunnel: w314 -> [_ w387 _ _ _ _ _ _ _ _]
          tunnel: w303 -> [_ _ w459 w615 _ _ _ _ _ _]
          tunnel: w313 -> [_ _ _ _ _ _ _ _ _ _]
          tunnel: w312 -> [_ w415 _ _ _ _ _ w946 _ _]
          tunnel: [_ w416 _ _ _ _ _ _ _ _] -> w310
          tunnel: [_ _ w453 _ _ _ _ _ _ _] -> w311
          tunnel: [_ _ w446 _ _ _ _ _ _ _] -> w309
          tunnel: [_ _ _ _ w687 _ _ _ _ _] -> w287
          tunnel: w305 -> [_ _ _ _ _ w806 _ _ _ _]
          tunnel: w306 -> [_ _ _ _ _ w807 _ _ _ _]
          tunnel: w304 -> [_ _ _ w616 _ _ _ _ _ _]
          tunnel: [_ _ _ w611 _ _ _ _ _ _] -> w289
          tunnel: w302 -> [_ w409 _ _ _ _ _ _ _ _]
          tunnel: w301 -> [_ w408 _ _ _ _ _ w945 _ _]
          tunnel: [_ w406 _ _ _ _ _ _ _ _] -> w300
          tunnel: [_ _ _ _ _ w805 _ _ _ _] -> w291
          tunnel: [_ _ _ _ _ w804 _ _ _ _] -> w293
          tunnel: w299 -> [_ w392 _ _ _ _ _ w933 _ _]
          tunnel: [_ w388 _ _ _ _ _ _ _ _] -> w298
          tunnel: [_ _ _ _ _ _ _ _ w966 _] -> w276
          tunnel: w275 -> [_ _ _ _ _ _ _ _ w961 _]
          tunnel: [_ _ _ _ _ _ _ _ w959 _] -> w274
          tunnel: w272 -> [_ _ _ _ _ _ _ _ _ w1036]
          tunnel: [_ _ _ _ _ _ _ _ _ w1035] -> w271
          tunnel: w270 -> [_ w386 _ _ _ _ _ _ _ _]
          tunnel: [_ w382 _ _ _ _ _ _ _ _] -> w269
          tunnel: w268 -> [_ _ w456 _ _ _ _ _ _ _]
          tunnel: w267 -> [_ _ w458 w608 _ _ _ w889 _ _]
          tunnel: [_ _ w442 _ _ _ _ _ _ _] -> w266
          frame #0 {
            # "CAEN channel names\nupdater, real-time"
            # "Also, dumping ground for variables and controls that may be updated during run-time"
            # "CAEN needle gauges\nMin. and Max. ranges"
            # "To view documentation of modules, look for icons that have a \"Descr.\" label near them,\nright-click these and select \"Description and tip\". For example on frame 2, \"High Voltage\",\na \"Quotient and Remainder\" icon on the left-hand side may be checked out, to view the\ndocumentation for the \"Reading Voltages and Currents\" module, which uses that icon. \n\nIf all else fails, consult the user manual, National Instruments knowledge base or Google."
            # "Time to wait, in between cycles"
            # "If the program is stopped, a final cycle executes without delay."
            # "Waiting for \"interval time\" to have passed, to start new cycle"
            n71 = call "Is Value Changed.vim"("value"="Channel Names (CAEN)") -> ("changed or first call?"=w334:bool)
            n72 = case shown="True" w334 {
              tunnel: "Channel Names (CAEN)" -> [_ w348]
              frame False {
              }
              frame True {
                n73 = Index Array(array=w348) -> (element #1=→"CAEN 1.0":string, element #2=→"CAEN 1.1":string, element #3=→"CAEN 1.2":string, element #4=→"CAEN 1.3":string, element #5=→"CAEN 2.0":string, element #6=→"CAEN 2.1":string, element #7=→"CAEN 2.2 2":string, element #8=→"CAEN 2.3 2":string)  [unwired: 8 in]
                "CAEN Ch. Names" <- w348
                "Channel Names" <- w348
                "Channel Names" <- w348
              }
            }
            n74 = Increment(x=w331) -> (x+1=w342:i32)
            n75 = local read "Channel Names (9207, ai0:7)"() -> (w332:string[])
            n76 = To Long Integer(number="Detector pressure input:") -> (32bit integer=→"Det.P input #":i32)
            n77 = To Long Integer(number="Flow meter input:") -> (32bit integer=→"Flow input #":i32)
            n78 = call "Is Value Changed.vim"("value"=w332) -> ("changed or first call?"=w333:bool)
            n79 = case shown="True" w333 {
              tunnel: w332 -> [_ w344]
              frame False {
                # ":D"
              }
              frame True {
                n80 = for {
                  tunnel: w344 -> [w347] mode=indexing
                  tunnel: [w345] -> w343 mode=indexing
                  i -> [w346]
                  n81 = Bundle("Or give name if \"Other\""=w347, w346) -> (w345:cluster{"Or give name if \"Other\"":string, i32})  [unwired: 1 in]
                }
                n82 = property on="Detector pressure input:" class="Ring (strict)"("StringsAndValues[]"=w343) -> ()  [unwired: 2 in, 2 out]
                n83 = property on="Flow meter input:" class="Ring (strict)"("StringsAndValues[]"=w343) -> ()  [unwired: 2 in, 2 out]
              }
            }
            n84 = case shown="False" w341 {
              tunnel: "Time per cycle (s)" -> [w373 _]
              frame False {
                n85 = while {
                  tunnel: w373 -> [w375]
                  stop <- w377 stop-if-true
                  n86 = call "Elapsed Time"("Time Target (s)"=w375) -> ("Elapsed Time (s)"=w376:dbl, "Time has Elapsed"=w377:bool)  [unwired: 11 in, 6 out]
                  n87 = Subtract(x=w375, y=w376) -> (x-y=→"Time until next cycle":dbl)
                }
              }
              frame True {
              }
            }
            n88 = stacked-sequence {
              frame #0 {
                n89 = property on="CAEN 1.0" class="Knob (strict)"("Scale.Minimum"="Scale.Range:Minimum", "Scale.Maximum"="Scale.Range:Maximum") -> ()  [unwired: 2 in, 2 out]
                n90 = property on="CAEN 1.1" class="Knob (strict)"("Scale.Minimum"="Scale.Range:Minimum 2", "Scale.Maximum"="Scale.Range:Maximum 2") -> ()  [unwired: 2 in, 2 out]
              }
              frame #1 {
                n91 = property on="CAEN 1.2" class="Knob (strict)"("Scale.Minimum"="Scale.Range:Minimum 3", "Scale.Maximum"="Scale.Range:Maximum 3") -> ()  [unwired: 2 in, 2 out]
                n92 = property on="CAEN 1.3" class="Knob (strict)"("Scale.Maximum"="Scale.Range:Maximum 4", "Scale.Minimum"="Scale.Range:Minimum 4") -> ()  [unwired: 2 in, 2 out]
              }
              frame #2 {
                n93 = property on="CAEN 2.1" class="Knob (strict)"("Scale.Maximum"="Scale.Range:Maximum 6", "Scale.Minimum"="Scale.Range:Minimum 6") -> ()  [unwired: 2 in, 2 out]
                n94 = property on="CAEN 2.0" class="Knob (strict)"("Scale.Maximum"="Scale.Range:Maximum 5", "Scale.Minimum"="Scale.Range:Minimum 5") -> ()  [unwired: 2 in, 2 out]
              }
              frame #3 {
                n95 = property on="CAEN 2.2" class="Knob (strict)"("Scale.Maximum"="Scale.Range:Maximum 7", "Scale.Minimum"="Scale.Range:Minimum 7") -> ()  [unwired: 2 in, 2 out]
                n96 = property on="CAEN 2.3" class="Knob (strict)"("Scale.Maximum"="Scale.Range:Maximum 8", "Scale.Minimum"="Scale.Range:Minimum 8") -> ()  [unwired: 2 in, 2 out]
              }
            }
            "Cycle number" <- w331
          }
          frame #1 {
            # "Module 3 tasks + status"
            # "Module 0, 1 tasks + status"
            # "Lake Shore task + status"
            # "Descr"
            # "NI 9207 8x V, 8x mA"
            # "Module 2 tasks+status"
            # "Temps (NI)"
            # "9216 T     (NI) x16\n9207 V     (NI)  x8\n9207 mA (NI)  x8\nTemp        (LS)  x2\nHeater %           x1"
            # "Temp A, Temp B, heater power"
            # "Measurements and conversions"
            n97 = stacked-sequence {
              tunnel: [w426] -> w416
              tunnel: w415 -> [w425]
              tunnel: [w424] -> w412
              tunnel: [w423] -> w411
              tunnel: [w422] -> w410
              tunnel: w409 -> [w420]
              tunnel: ["Setpoint (°C)"] -> w407
              frame #0 {
                # "LS output"
                # "P\nI\nD"
                n98 = Select(t=0, s=w420, f="Heater range") -> (s? t:f=w417:i32)
                "Heater Range" <- w417
                n99 = Unbundle("PID settings") -> ("P"=w431:dbl, "I"=w430:dbl, "D"=w429:dbl)
                n100 = Unbundle(w425) -> ("VISA resource name out"=w433:refnum<visa-resource-name>, "error out"=w432:errorcluster)
                n101 = call "Lakeshore subVI.vi"("Setpoint"="Setpoint (°C)", "Rate (D) (X.X %)"=w429, "Range"=w417, "Reset (I) (XX.X)"=w430, "Gain (P) (XX.X)"=w431, "error in (no error)"=w432, "VISA resource name"=w433) -> ("Input B"=w423:dbl, "Input A"=w424:dbl, "error out"=w427:errorcluster, "VISA resource name out"=w428:refnum<visa-resource-name>, "Heater 1 (%)"=w422:dbl)
                "Lakeshore" <- w427
                n102 = Bundle("VISA resource name out"=w428, "error out"=w427) -> (w426:T6)  [unwired: 1 in]
              }
            }
            n103 = Get Date/Time In Seconds() -> (seconds since 1Jan1904=w414:timestamp)
            n104 = Unbundle(w392) -> ("task out"=w391:refnum<k21>, "error out"=w390:errorcluster)
            n105 = Build Array (concatenate)(w387, w414) -> (w413:timestamp[])
            n106 = Unbundle(w408) -> ("task out"=w397:refnum<k21>, "error out"=w396:errorcluster)
            n107 = call-poly <vilib>:"DAQmx Read.vi"("task/channels in"=w391, "error in"=w390) -> ("task out"=w380:refnum<k21>, "data"=w378:dbl[], "error out"=w389:errorcluster)  [unwired: 11 in]
            "PT100 data" <- w378
            "NI 9216 x2" <- w389
            n108 = call-poly <vilib>:"DAQmx Read.vi"("task/channels in"=w397, "error in"=w396) -> ("task out"=w395:refnum<k21>, "data"=w404:dbl[], "error out"=w394:errorcluster)  [unwired: 11 in]
            "Raw readouts (V, mA)" <- w404
            "NI 9207" <- w394
            n109 = Build Array (concatenate)("Offsets\nsubtracted", "Offsets\nsubtracted") -> (w398:dbl[])
            n110 = Build Array (concatenate)("Multipliers", "Multipliers") -> (w401:dbl[])
            n111 = for {
              tunnel: w398 -> [w439] mode=indexing
              tunnel: w404 -> [w438] mode=indexing
              tunnel: w401 -> [w436] mode=indexing
              tunnel: [w435] -> w405 mode=indexing
              n112 = Subtract(x=w438, y=w439) -> (x-y=w437:dbl)
              n113 = Multiply(x=w437, y=w436) -> (x*y=w435:dbl)
            }
            n114 = Bundle("task out"=w380, "error out"=w389) -> (w388:T5)  [unwired: 1 in]
            n115 = Bundle("task out"=w395, "error out"=w394) -> (w406:T5)  [unwired: 1 in]
            n116 = Build Array(w412, w411, w410) -> (w393:dbl[])
            "LakeShore readings" <- w393
            n117 = Unbundle(w386) -> ("task out"=w379:refnum<k21>, "error out"=w385:errorcluster)
            n118 = call-poly <vilib>:"DAQmx Read.vi"("task/channels in"=w379, "error in"=w385) -> ("task out"=w384:refnum<k21>, "data"=w381:dbl[], "error out"=w383:errorcluster)  [unwired: 11 in]
            "NI 9226" <- w383
            "PT1000 data" <- w381
            n119 = Bundle("task out"=w384, "error out"=w383) -> (w382:T5)  [unwired: 1 in]
          }
          frame #2 {
            # "Alter voltages if button clicked"
            # "Descr."
            # "VMON1  x4 \nVMON2  x4\nIMON1    x4\nIMON2    x4"
            # "Needle gauge Voltage displays"
            # "High Voltage"
            n120 = for {
              tunnel: w459 -> [w607] mode=indexing
              tunnel: w458 -> [w606] mode=indexing
              tunnel: [w605] -> w451 mode=indexing
              tunnel: [w604] -> w450 mode=indexing
              tunnel: [w603] -> w457 mode=concatenating
              tunnel: [w602] -> w454 mode=concatenating
              n121 = call "Read_supply_with_boardhandle.vi"("error in (no error)"=w606, "BoardHandle"=w607) -> ("error out"=w604:errorcluster, "IMon values (uA)"=w602:dbl[], "VMon values (V)"=w603:dbl[], "BoardHandle out"=w605:T8)  [unwired: 6 in]
            }
            "IMon (uA)" <- w454
            n122 = Build Array (concatenate)("VSet (V)", "VMax (V)", "IMax (uA)") -> (w469:dbl[])
            n123 = case shown="True" "Query HV status" {
              tunnel: w451 -> [w585 w593]
              tunnel: w450 -> [w584 w592]
              tunnel: [w585 w587] -> w448
              tunnel: [w584 w586] -> w447
              frame False {
              }
              frame True {
                n124 = for {
                  tunnel: w593 -> [w598] mode=indexing
                  tunnel: w592 -> [w597] mode=indexing
                  tunnel: [w596] -> w587 mode=indexing
                  tunnel: [w595] -> w586 mode=indexing
                  tunnel: [w594] -> w591 mode=concatenating
                  n125 = call <instrlib>:"Channel Status.vi"("error in (no error)"=w597, "BoardHandle"=w598) -> ("error out"=w595:errorcluster, "Channel Status Array"=w594:T2, "BoardHandle out"=w596:T4)  [unwired: 7 in]
                }
                n126 = Delete From Array(array=w591, length=4) -> (deleted portion=→"CAEN 1":T2, array with subset deleted=→"CAEN 2":T2)  [unwired: 1 in]
              }
            }
            n127 = Or(x="Kill all channels (Trip)", y="Kill voltage") -> (x .or. y?=w460:bool)
            n128 = for {
              tunnel: w457 -> [w600] mode=indexing
              tunnel: w456 -> [w601] mode=indexing
              tunnel: [w599] -> w455 mode=indexing
              n129 = Multiply(x=w601, y=w600) -> (x*y=w599:dbl)
            }
            "Voltages" <- w455
            "Vmon (V)" <- w455
            n130 = Build Array("Apply Voltage", "Set to zero (ramp down)", w460) -> (w465:bool[])
            n131 = Build Array (concatenate)(w455, w454) -> (w453:dbl[])
            n132 = Search 1D Array(1D array=w465, element=TRUE) -> (index of element=w449:i32)  [unwired: 1 in]
            n133 = case shown="2" w449 {
              tunnel: w448 -> [w498 w533 w567 w583]
              tunnel: w447 -> [w497 w532 w566 w582]
              tunnel: [w479 w517 w551 w583] -> w446
              tunnel: [w476 w514 w548 w582] -> w442
              tunnel: "VSet (V)" -> [w495 _ w564 _]
              tunnel: "VMax (V)" -> [w494 w530 _ _]
              tunnel: "IMax (uA)" -> [w493 w529 w563 _]
              frame 0 {
                w492 = 4 ("length")
                # "Split up arrays"
                # "Apply settings"
                n134 = Delete From Array(array=w494, length=w492) -> (deleted portion=w483:u16[], array with subset deleted=w490:u16[])  [unwired: 1 in]
                n135 = Delete From Array(array=w493, length=w492) -> (deleted portion=w482:sgl[], array with subset deleted=w489:sgl[])  [unwired: 1 in]
                n136 = Delete From Array(array=w495, length=w492) -> (deleted portion=w484:dbl[], array with subset deleted=w491:dbl[])  [unwired: 1 in]
                n137 = Index Array(array=w498) -> (element #1=w488:T4, element #2=w486:T4)  [unwired: 2 in]
                n138 = Index Array(array=w497) -> (element #1=w487:errorcluster, element #2=w485:errorcluster)  [unwired: 2 in]
                n139 = for {
                  N: 4 -> [_]
                  tunnel: w491 -> [w510] mode=indexing
                  tunnel: w490 -> [w509] mode=indexing
                  tunnel: w489 -> [w508] mode=indexing
                  tunnel: w488 -> [w512]
                  tunnel: w487 -> [w511]
                  tunnel: w486 -> [w507]
                  tunnel: w485 -> [w506]
                  tunnel: w484 -> [w505] mode=indexing
                  tunnel: w483 -> [w504] mode=indexing
                  tunnel: w482 -> [w503] mode=indexing
                  tunnel: [w502] -> w481
                  tunnel: [w501] -> w478
                  tunnel: [w500] -> w480
                  tunnel: [w499] -> w477
                  i -> [w513]
                  n140 = call "Set_supply_with_boardhandle.vi"("Current Limit (0.00 uA)"=w503, "Channel (0)"=w513, "error in (no error)"=w506, "Voltage Max (0.0 V)"=w504, "Voltage Level (0.0 V)"=w505, "BoardHandle"=w507) -> ("error out"=w499:errorcluster, "BoardHandle out"=w500:T8)  [unwired: 4 in]
                  n141 = call "Set_supply_with_boardhandle.vi"("Current Limit (0.00 uA)"=w508, "Channel (0)"=w513, "error in (no error)"=w511, "Voltage Max (0.0 V)"=w509, "Voltage Level (0.0 V)"=w510, "BoardHandle"=w512) -> ("error out"=w501:errorcluster, "BoardHandle out"=w502:T8)  [unwired: 4 in]
                }
                n142 = Build Array(w481, w480) -> (w479:T7)
                n143 = Build Array(w478, w477) -> (w476:errorcluster[])
              }
              frame 1 {
                w528 = 4 ("length")
                # "Split up arrays"
                # "Set VSet to zero"
                n144 = Delete From Array(array=w530, length=w528) -> (deleted portion=w521:u16[], array with subset deleted=w527:u16[])  [unwired: 1 in]
                n145 = Delete From Array(array=w529, length=w528) -> (deleted portion=w520:sgl[], array with subset deleted=w526:sgl[])  [unwired: 1 in]
                n146 = Index Array(array=w533) -> (element #1=w525:T4, element #2=w523:T4)  [unwired: 2 in]
                n147 = Index Array(array=w532) -> (element #1=w524:errorcluster, element #2=w522:errorcluster)  [unwired: 2 in]
                n148 = for {
                  N: 4 -> [_]
                  tunnel: w527 -> [w544] mode=indexing
                  tunnel: w526 -> [w543] mode=indexing
                  tunnel: w525 -> [w546]
                  tunnel: w524 -> [w545]
                  tunnel: w523 -> [w542]
                  tunnel: w522 -> [w541]
                  tunnel: w521 -> [w540] mode=indexing
                  tunnel: w520 -> [w539] mode=indexing
                  tunnel: [w538] -> w519
                  tunnel: [w537] -> w516
                  tunnel: [w536] -> w518
                  tunnel: [w535] -> w515
                  i -> [w547]
                  w534 = 0
                  n149 = call "Set_supply_with_boardhandle.vi"("Current Limit (0.00 uA)"=w539, "Channel (0)"=w547, "error in (no error)"=w541, "Voltage Max (0.0 V)"=w540, "Voltage Level (0.0 V)"=w534, "BoardHandle"=w542) -> ("error out"=w535:errorcluster, "BoardHandle out"=w536:T8)  [unwired: 4 in]
                  n150 = call "Set_supply_with_boardhandle.vi"("Current Limit (0.00 uA)"=w543, "Channel (0)"=w547, "error in (no error)"=w545, "Voltage Max (0.0 V)"=w544, "Voltage Level (0.0 V)"=w534, "BoardHandle"=w546) -> ("error out"=w537:errorcluster, "BoardHandle out"=w538:T8)  [unwired: 4 in]
                }
                n151 = Build Array(w519, w518) -> (w517:T7)
                n152 = Build Array(w516, w515) -> (w514:errorcluster[])
              }
              frame 2 {
                w562 = 4 ("length")
                # "Split up arrays"
                # "Kill voltage (make all channels Trip)"
                n153 = Delete From Array(array=w563, length=w562) -> (deleted portion=w554:sgl[], array with subset deleted=w560:sgl[])  [unwired: 1 in]
                n154 = Delete From Array(array=w564, length=w562) -> (deleted portion=w555:dbl[], array with subset deleted=w561:dbl[])  [unwired: 1 in]
                n155 = Index Array(array=w567) -> (element #1=w559:T4, element #2=w557:T4)  [unwired: 2 in]
                n156 = Index Array(array=w566) -> (element #1=w558:errorcluster, element #2=w556:errorcluster)  [unwired: 2 in]
                n157 = for {
                  N: 4 -> [_]
                  tunnel: w561 -> [w578] mode=indexing
                  tunnel: w560 -> [w577] mode=indexing
                  tunnel: w559 -> [w580]
                  tunnel: w558 -> [w579]
                  tunnel: w557 -> [w576]
                  tunnel: w556 -> [w575]
                  tunnel: w555 -> [w574] mode=indexing
                  tunnel: w554 -> [w573] mode=indexing
                  tunnel: [w572] -> w553
                  tunnel: [w571] -> w550
                  tunnel: [w570] -> w552
                  tunnel: [w569] -> w549
                  i -> [w581]
                  w568 = 0
                  n158 = call "Set_supply_with_boardhandle.vi"("Current Limit (0.00 uA)"=w573, "Channel (0)"=w581, "error in (no error)"=w575, "Voltage Max (0.0 V)"=w568, "Voltage Level (0.0 V)"=w574, "BoardHandle"=w576) -> ("error out"=w569:errorcluster, "BoardHandle out"=w570:T8)  [unwired: 4 in]
                  n159 = call "Set_supply_with_boardhandle.vi"("Current Limit (0.00 uA)"=w577, "Channel (0)"=w581, "error in (no error)"=w579, "Voltage Max (0.0 V)"=w568, "Voltage Level (0.0 V)"=w578, "BoardHandle"=w580) -> ("error out"=w571:errorcluster, "BoardHandle out"=w572:T8)  [unwired: 4 in]
                }
                n160 = Build Array(w553, w552) -> (w551:T7)
                n161 = Build Array(w550, w549) -> (w548:errorcluster[])
              }
              frame 3, Default {
                # "Do nothing"
              }
            }
            n162 = Index Array(array=w453) -> (element #1=→"CAEN 1.0":dbl, element #2=→"CAEN 1.1":dbl, element #3=→"CAEN 1.2":dbl, element #4=→"CAEN 1.3":dbl, element #5=→"CAEN 2.0":dbl, element #6=→"CAEN 2.1":dbl, element #7=→"CAEN 2.2":dbl, element #8=→"CAEN 2.3":dbl)  [unwired: 8 in]
            n163 = Index Array(array=w442) -> (element #1=→"CAEN 1":errorcluster, element #2=→"CAEN 2":errorcluster)  [unwired: 2 in]
          }
          frame #3 {
            # "Descr."
            # "Reset anode"
            n164 = Or Array Elements(Boolean array=w610) -> (logical OR=w609:bool)
            n165 = case shown="True" "Reset anode\nperiodically?" {
              tunnel: w616 -> [_ w625]
              tunnel: w615 -> [_ w632]
              tunnel: w614 -> [_ w637]
              tunnel: w609 -> [_ w623]
              tunnel: [w617 w624] -> w611
              tunnel: w608 -> [_ w621]
              frame False {
                # "Anode Reset Routine inactive:\nkeep timers up to date so activating\nroutine will correctly initiate the timers."
                n166 = Get Date/Time In Seconds() -> (seconds since 1Jan1904=w619:timestamp)
                n167 = To Double Precision Float(number=w619) -> (double precision float=w618:dbl)
                n168 = Build Array(w618, w618) -> (w617:dbl[])
              }
              frame True {
                n169 = case shown="\"CAEN 1\", Default" "CAEN unit selector" {
                  tunnel: w632 -> [w652 w658]
                  tunnel: [0 4] -> w630
                  tunnel: [w650 w656] -> w622
                  tunnel: w621 -> [w649 w654]
                  tunnel: [w648 w653] -> w620
                  frame "CAEN 1", Default {
                    n170 = Index Array(array=w652) -> (element=w650:T4)  [unwired: 1 in]
                    n171 = Index Array(array=w649) -> (element=w648:errorcluster)  [unwired: 1 in]
                  }
                  frame "CAEN 2" {
                    n172 = Index Array(array=w658, index=1) -> (element=w656:T4)
                    n173 = Index Array(array=w654, index=1) -> (element=w653:errorcluster)
                  }
                }
                n174 = call "anode_timing.vi"("Keep off for X seconds"="Keep off for X seconds", "Array of timers"=w625, "Kill every Y minutes"="Kill every Y minutes") -> ("Time to kill"=w639:bool, "Time until reset"=→"Seconds until \nanode reset":dbl, "Time until autokill"=→"Seconds until \nanode autokill":dbl, "Time to reset"=w640:bool)  [unwired: 5 in]
                "Killed" <- w639
                "Restarted" <- w640
                n175 = Add(x=w630, y="Anode ch.") -> (x+y=w628:i32)
                n176 = Build Array(w639, w640, w623) -> (w643:bool[])
                n177 = Add(x=w628, y=8) -> (x+y=w633:i32)
                n178 = Add(x=w628, y=16) -> (x+y=w634:i32)
                n179 = Search 1D Array(1D array=w643, element=TRUE) -> (index of element=w642:i32)  [unwired: 1 in]
                n180 = Index Array(array=w637, index #1=w628, index #2=w633, index #3=w634) -> (element #1=w646:dbl, element #2=w644:dbl, element #3=w645:dbl)
                n181 = case shown="0" w642 {
                  tunnel: w646 -> [_ w674 _ _]
                  tunnel: w644 -> [w666 w675 _ _]
                  tunnel: w645 -> [w665 w676 _ _]
                  tunnel: "Anode ch." -> [w662 w677 _ _]
                  tunnel: w625 -> [w668 _ _ w686]
                  tunnel: [w667 w680 w683 w686] -> w624
                  tunnel: w622 -> [w663 w678 _ _]
                  tunnel: w620 -> [w664 w679 _ _]
                  frame 0 {
                    # "Set Anode Voltage to zero,\nreset the 1st timer"
                    # "Anode Vset to zero"
                    n182 = Get Date/Time In Seconds() -> (seconds since 1Jan1904=w671:timestamp)
                    n183 = call "Set_supply_with_boardhandle.vi"("Current Limit (0.00 uA)"=w665, "Channel (0)"=w662, "error in (no error)"=w664, "Voltage Max (0.0 V)"=w666, "Voltage Level (0.0 V)"=0, "BoardHandle"=w663) -> ("error out"=w661:errorcluster)  [unwired: 4 in, 1 out]
                    n184 = Index Array(array=w668, index=1) -> (element=w669:dbl)
                    n185 = To Double Precision Float(number=w671) -> (double precision float=w670:dbl)
                    n186 = Build Array(w670, w669) -> (w667:dbl[])
                    n187 = call <vilib>:"Simple Error Handler.vi"("error in (no error)"=w661) -> ()  [unwired: 4 in, 5 out]
                  }
                  frame 1 {
                    # "Set Anode Voltage to defined value,\nreset both timers"
                    # "Anode Vset applied"
                    n188 = Get Date/Time In Seconds() -> (seconds since 1Jan1904=w682:timestamp)
                    n189 = call "Set_supply_with_boardhandle.vi"("Current Limit (0.00 uA)"=w676, "Channel (0)"=w677, "error in (no error)"=w679, "Voltage Max (0.0 V)"=w675, "Voltage Level (0.0 V)"=w674, "BoardHandle"=w678) -> ("error out"=w673:errorcluster)  [unwired: 4 in, 1 out]
                    n190 = To Double Precision Float(number=w682) -> (double precision float=w681:dbl)
                    n191 = Build Array(w681, w681) -> (w680:dbl[])
                    n192 = call <vilib>:"Simple Error Handler.vi"("error in (no error)"=w673) -> ()  [unwired: 4 in, 5 out]
                  }
                  frame 2 {
                    # "Change Voltage button pressed"
                    # "Reset both timers"
                    n193 = Get Date/Time In Seconds() -> (seconds since 1Jan1904=w685:timestamp)
                    n194 = To Double Precision Float(number=w685) -> (double precision float=w684:dbl)
                    n195 = Build Array(w684, w684) -> (w683:dbl[])
                  }
                  frame 3, Default {
                    # "Timers stay at previous value,\nso difference between those and\ncurrent time keeps incrementing"
                    # "No event"
                  }
                }
              }
            }
            n196 = To Time Stamp(1:w611) -> (0:→"Anode timers":timestamp[])
            "?" <- "Reset anode\nperiodically?"
          }
          frame #4 {
            # "Det. P"
            # "Flow"
            # "Flexibly acquire indices"
            # "Plots 9207 output vs time"
            # "Descr."
            # "Moving averages"
            # "Historic graphs: Phase, 9207 ai, Flow, Heater, Temperature"
            # "Non-historic Temperature + Det. Pressure"
            # "Updated TOBA >>>"
            # "Descr."
            # "Latest Detector Pressure"
            # "Plots individual lists of Temp. vs. t"
            # "Plots and moving averages"
            n197 = Build Array (concatenate)(w712, w698, w709, w711) -> (w740:dbl[])
            n198 = Build Array (concatenate)(w741, w740) -> (w696:dbl[][])
            n199 = Array Size(array=w709) -> (size(s)=w708:i32)
            n200 = Array Size(array=w698) -> (size(s)=w710:i32)
            n201 = Array Size(array=w712) -> (size(s)=w699:i32)
            n202 = Add(x=w699, y=w710) -> (x+y=w694:i32)
            n203 = Add(x=w694, y=w708) -> (x+y=w707:i32)
            n204 = local read "Flow input #"() -> (w718:i32)
            n205 = local read "Det.P input #"() -> (w719:i32)
            n206 = Add(x=w707, y=2 ("disabled index (col)")) -> (x+y=w705:i32)
            n207 = Equal?(x=666, y="Temperature channel selector") -> (x = y?=w734:bool)
            n208 = Index Array(array=w696, index (col)=w705) -> (element=w704:dbl[])  [unwired: 1 in]
            n209 = case shown="True" w734 {
              tunnel: w698 -> [w779 w780]
              tunnel: [w778 w781] -> w732
              tunnel: "Temperature channel selector" -> [w777 _]
              frame False {
                n210 = Index Array(array=w779, index=w777) -> (element=w778:dbl)
              }
              frame True {
                n211 = Add Array Elements(numeric array=w780) -> (sum=w782:dbl)
                n212 = Array Size(array=w780) -> (size(s)=w783:i32)
                n213 = Divide(x=w782, y=w783) -> (x/y=w781:dbl)
              }
            }
            n214 = Add(x=w719, y=w694) -> (x+y=w728:i32)
            n215 = Add(x=w694, y=w718) -> (x+y=w726:i32)
            n216 = Bundle(w687, w704) -> (w701:cluster{timestamp[], dbl[]})  [unwired: 1 in]
            n217 = Build Array(w701) -> (→"Heater power (%)":cluster{timestamp[], dbl[]}[])
            n218 = Add(x=w699, y="Temperature Channel Selector") -> (x+y=w702:i32)
            n219 = Index Array(array=w696, index (col) #1=w728, index (col) #2=w726) -> (element #1=w727:dbl[], element #2=w716:dbl[])  [unwired: 2 in]
            n220 = local read "Det.P input #"() -> (w720:i32)
            n221 = Index Array(array=w696, index (col)=w702) -> (element=w731:dbl[])  [unwired: 1 in]
            n222 = for {
              N: 8 -> [_]
              tunnel: w696 -> [w770]
              tunnel: w687 -> [w763]
              tunnel: [w767] -> w724 mode=indexing
              tunnel: [w762] -> w723 mode=indexing
              tunnel: w694 -> [w760]
              i -> [w766]
              n223 = Add(x=w760, y=8) -> (x+y=w759:i32)
              n224 = Add(x=w760, y=w766) -> (x+y=w769:i32)
              n225 = Add(x=w766, y=w759) -> (x+y=w765:i32)
              n226 = Index Array(array=w770, index (col) #1=w769, index (col) #2=w765) -> (element #1=w768:dbl[], element #2=w764:dbl[])  [unwired: 2 in]
              n227 = Bundle(w763, w768) -> (w767:cluster{timestamp[], dbl[]})  [unwired: 1 in]
              n228 = Bundle(w763, w764) -> (w762:cluster{timestamp[], dbl[]})  [unwired: 1 in]
            }
            "9207 (ai 0:7, Volts)" <- w724
            "9207 (ai 8:15, Amperes)" <- w723
            n229 = Bundle(w731, w727) -> (w745:cluster{dbl[], dbl[]})  [unwired: 1 in]
            n230 = Index Array(array=w709, index=w720) -> (element=w746:dbl)
            n231 = call "moving_avg.vi"("N samples"="N samples", "Array"=w727) -> ("Numeric"=→"Detector Pressure":dbl)  [unwired: 9 in]
            n232 = call "moving_avg.vi"("N samples"="N samples", "Array"=w716) -> ("Numeric"=→"Average Flow (SLPM)":dbl)  [unwired: 9 in]
            n233 = Bundle(w687, w716) -> (w743:cluster{timestamp[], dbl[]})  [unwired: 1 in]
            n234 = Build Array(w745) -> (→"Historical Large Phase Diagram":cluster{dbl[], dbl[]}[])
            n235 = Bundle("Waveform"=w732, w746) -> (w750:cluster{"Waveform":dbl, dbl})  [unwired: 1 in]
            n236 = Build Array(w743) -> (→"Flow (SLPM)":cluster{timestamp[], dbl[]}[])
            n237 = Build Array(w750) -> (→"Phase Diagram":cluster{"Waveform":dbl, dbl}[])
            n238 = for {
              N: w699 -> [_]
              tunnel: w687 -> [w795]
              tunnel: [w794] -> w751 mode=indexing
              tunnel: w696 -> [w793]
              i -> [w791]
              n239 = Index Array(array=w793, index (col)=w791) -> (element=w792:dbl[])  [unwired: 1 in]
              n240 = Bundle(w795, w792) -> (w794:cluster{timestamp[], dbl[]})  [unwired: 1 in]
            }
            "Setup Temperature (9216 0:15, °C)" <- w751
            n241 = Increment(x=w694) -> (x+1=w695:i32)
            n242 = Array Size(array=w698) -> (size(s)=w697:i32)
            n243 = Equal?(x=666, y="Temperature Channel Selector") -> (x = y?=w736:bool)
            n244 = Index Array(array=w696, index (col) #1=w694, index (col) #2=w695) -> (element #1=w693:dbl[], element #2=w692:dbl[])  [unwired: 2 in]
            n245 = local read "Channel Names (9207, ai0:7)"() -> (w721:string[])
            n246 = local read "Channel Names (9207, ai8:15)"() -> (w722:string[])
            n247 = case shown="False" w736 {
              tunnel: w698 -> [w786 w787]
              tunnel: [w785 w788] -> w739
              tunnel: "Temperature Channel Selector" -> [w784 _]
              frame False {
                n248 = Index Array(array=w786, index=w784) -> (element=w785:dbl)
              }
              frame True {
                n249 = Add Array Elements(numeric array=w787) -> (sum=w789:dbl)
                n250 = Array Size(array=w787) -> (size(s)=w790:i32)
                n251 = Divide(x=w789, y=w790) -> (x/y=w788:dbl)
              }
            }
            n252 = for {
              N: w697 -> [_]
              tunnel: w687 -> [w758]
              tunnel: [w757] -> w691 mode=indexing
              tunnel: w696 -> [w756]
              tunnel: w699 -> [w752]
              i -> [w753]
              n253 = Add(x=w752, y=w753) -> (x+y=w754:i32)
              n254 = Index Array(array=w756, index (col)=w754) -> (element=w755:dbl[])  [unwired: 1 in]
              n255 = Bundle(w758, w755) -> (w757:cluster{timestamp[], dbl[]})  [unwired: 1 in]
            }
            n256 = Bundle(w687, w693) -> (w690:cluster{timestamp[], dbl[]})  [unwired: 1 in]
            n257 = Bundle(w687, w692) -> (w689:cluster{timestamp[], dbl[]})  [unwired: 1 in]
            n258 = call "Is Value Changed.vim"("value"=w722) -> ("changed or first call?"=w729:bool)
            n259 = call "Is Value Changed.vim"("value"=w721) -> ("changed or first call?"=w730:bool)
            n260 = case shown="True" w729 {
              tunnel: w722 -> [_ w771]
              frame False {
              }
              frame True {
                n261 = for {
                  tunnel: w771 -> [w772] mode=indexing
                  i -> [w773]
                  n262 = property on="9207 (ai 8:15, Amperes)" class="XYGraph (strict)"("Active Plot"=w773, "Plot.Plot Name"=w772) -> ()  [unwired: 2 in, 2 out]
                }
              }
            }
            n263 = case shown="True" w730 {
              tunnel: w721 -> [_ w774]
              frame False {
              }
              frame True {
                n264 = for {
                  tunnel: w774 -> [w775] mode=indexing
                  i -> [w776]
                  n265 = property on="9207 (ai 0:7, Volts)" class="XYGraph (strict)"("Active Plot"=w776, "Plot.Plot Name"=w775) -> ()  [unwired: 2 in, 2 out]
                }
              }
            }
            n266 = Bundle("Waveform"=w739, w746) -> (w748:cluster{"Waveform":dbl, dbl})  [unwired: 1 in]
            n267 = Build Array (concatenate)(w691, w690, w689) -> (→"Low Temperature (9226 0:7 and LakeShore A;B, °C)":cluster{timestamp[], dbl[]}[])
            n268 = Build Array(w748) -> (→"Large Phase Diagram":cluster{"Waveform":dbl, dbl}[])
          }
          frame #5 {
            # "Temperatures x8\nTo indicators on schematic\ninside detector"
            # "Temp A, Temp B, Heater%"
            # "Temperatures x16\nTo indicators on the physical schematic"
            # "Individual latest 9207 readings.\nIndicators go here. Array is 1x16,\nitems have been converted using\nthe offsets and multipliers"
            # "Displays"
            n269 = local read "Flow input #"() -> (w801:i32)
            n270 = case shown="False" "Reset?" {
              tunnel: [w813 0.0] -> w809
              tunnel: w806 -> [w813 _]
              frame False {
              }
              frame True {
              }
            }
            n271 = Index Array(array=w800) -> ()  [unwired: 16 in, 16 out]
            n272 = Index Array(array=w800, index=w801) -> (element=w804:dbl)
            n273 = call "Average_flow_x_time.vi"("Array of timestamps"=w808, "Previous Flow"=w807, "Latest Flow"=w804) -> ("Volume (SL)"=w810:dbl)  [unwired: 8 in]
            n274 = case shown="False" "Pause?" {
              tunnel: w809 -> [w817 w818]
              tunnel: w810 -> [w816 _]
              tunnel: [w815 w818] -> w805
              frame False {
                n275 = Add(x=w816, y=w817) -> (x+y=w815:dbl)
              }
              frame True {
              }
            }
            "Integrated Flow (SL)" <- w805
            n276 = Index Array(array=w802) -> (element #1=→"Coldhead (°C)" →"Temp A":dbl, element #2=→"Heater (°C)" →"Temp B":dbl)  [unwired: 3 in, 1 out]
            n277 = Index Array(array=w803) -> ()  [unwired: 16 in, 16 out]
            n278 = Index Array(array=w796) -> ()  [unwired: 8 in, 8 out]
            "9207 (V; A) Converted" <- w800
            "9216 #1 (°C)" <- w803
            "9216 #2 (°C)" <- w803
            "Setpoint (°C)" <- w797
          }
          frame #6 {
            # "The same order applies to the headers resaved,\nbut with an additional line, stating the date/time"
            # "-----------DATA SAVED----------\nHuman-readable timestamp  ;\nTemperatures (16),  2xNI 9216;\nTemperatures (8),        NI 9226;\nVolts, Amps  (8 x2),     NI 9207;\nTemperature (2),    Lakeshore;\nHeater power (1),  Lakeshore;\nSetpoint (1),           Lakeshore;\nHV readouts (16)          CAEN ;\nCurrent time (s)                ---   ;\nCycle time (s)                    ---   ;"
            # "Saving data"
            n279 = Get Date/Time In Seconds() -> (seconds since 1Jan1904=w841:timestamp)
            n280 = To Double Precision Float(number=w841) -> (double precision float=w824:dbl)
            n281 = Build Array (concatenate)(w827, w819, w820, w821, w822, w823, w824, w825) -> (w840:dbl[])
            n282 = Array Size(array=w827) -> (size(s)=w828:i32)
            n283 = Array Size(array=w819) -> (size(s)=w829:i32)
            n284 = Add(x=w828, y=w829) -> (x+y=w826:i32)
            n285 = Get Date/Time String() -> (date string=w834:string)  [unwired: 3 in, 1 out]
            n286 = case shown="True" "Re-save headers" {
              tunnel: w826 -> [_ w842]
              frame False {
                # "Just sit around and feel pretty"
              }
              frame True {
                w850 = ""
                # "Append line of most recent channel names to header file"
                n287 = local read "Channel Names (CAEN)"() -> (w849:string[])
                n288 = local read "Channel Names (9207, ai0:7)"() -> (w857:string[])
                n289 = for {
                  N: w842 -> [_]
                  shift-right: [w881] -> w853
                  shift-left: "" -> [w882]
                  i -> [w886]
                  n290 = Format Into String(initial string="t", w886) -> (resulting string=w884:string)  [unwired: 2 in, 1 out]
                  n291 = Concatenate Strings(w882, w884, "\t") -> (w881:string)
                }
                n292 = for {
                  shift-right: [w879] -> w855
                  shift-left: w850 -> [w880]
                  tunnel: w857 -> [w877] mode=indexing
                  n293 = Concatenate Strings(w880, w877, "\t") -> (w879:string)
                }
                n294 = local read "Channel Names (9207, ai8:15)"() -> (w856:string[])
                n295 = for {
                  tunnel: w849 -> [w871] mode=indexing
                  shift-right: [w869] -> w844
                  shift-left: w850 -> [w868]
                  n296 = Concatenate Strings(w868, w871, " (V)", "\t") -> (w869:string)
                }
                n297 = for {
                  shift-right: [w875] -> w852
                  shift-left: w855 -> [w876]
                  tunnel: w856 -> [w873] mode=indexing
                  n298 = Concatenate Strings(w876, w873, "\t") -> (w875:string)
                }
                n299 = for {
                  tunnel: w849 -> [w866] mode=indexing
                  shift-right: [w864] -> w848
                  shift-left: w844 -> [w863]
                  n300 = Concatenate Strings(w863, w866, " (I)", "\t") -> (w864:string)
                }
                n301 = Get Date/Time String() -> (date string=w861:string)  [unwired: 3 in, 1 out]
                n302 = Format Date/Time String() -> (date/time string=w843:string)  [unwired: 3 in]
                n303 = Build Path(base path=path "D:/Log_data/SC_LOG_HEADERS", name or relative path=w861) -> (appended path=w860:path)
                n304 = Concatenate Strings("Time\t", w853, w852, "Temp A\tTemp B\tHeater Power\tSetpoint\t", w848, "Time in seconds\tTime per cycle\t", w843, "\r\n") -> (w845:string)
                n305 = call <vilib>:"Write Spreadsheet String.vi"("append to file? (new file:F)"=TRUE, "spreadsheet string"=w845, "file path (dialog if empty)"=w860) -> ()  [unwired: 7 in, 2 out]
              }
            }
            n306 = Build Path(base path=path "D:/Log_data/SC_LOG", name or relative path=w834) -> (appended path=w833:path)
            n307 = Format Date/Time String() -> (date/time string=w838:string)  [unwired: 3 in]
            n308 = Array To Spreadsheet String(array=w840, 3:"%.3f" ("format string")) -> (spreadsheet string=w836:string)  [unwired: 1 in]
            n309 = Concatenate Strings(w838, "\t", w836) -> (w832:string)
            n310 = call <vilib>:"Write Spreadsheet String.vi"("append to file? (new file:F)"=TRUE, "spreadsheet string"=w832, "file path (dialog if empty)"=w833) -> ()  [unwired: 7 in, 2 out]
          }
          frame #7 {
            # "Status is True if ANY (armed)\ncondition is met"
            # "Detector P. Alert"
            # "Uninteruptable\n Power Supply Alert"
            # "Temp. Warning"
            # "Arms"
            # "Comm. Alert"
            # "Temperature Alert"
            # "Alarm conditions (Temp)"
            # "Check Alarms and Warnings"
            n311 = Index Array(array=w889) -> (element #1=w888:errorcluster, element #2=w887:errorcluster)  [unwired: 2 in]
            n312 = Unbundle By Name(w933) -> ("error out.status"=w915:bool)
            "NI mod 2&3 status" <- w915
            n313 = Unbundle By Name(w945) -> ("error out.status"=w941:bool)
            "NI mod1 (P) status" <- w941
            n314 = Unbundle By Name(w946) -> ("error out.status"=w944:bool)
            "LakeShore status" <- w944
            n315 = Unbundle By Name(w887) -> ("status"=w942:bool)
            "CAEN 2 status" <- w942
            n316 = Unbundle By Name(w888) -> ("status"=w943:bool)
            "CAEN 1 status" <- w943
            n317 = Build Array(w944, w943, w942, w941, w915) -> (w916:bool[])
            n318 = Build Array("LakeShore", "CAEN 1", "CAEN 2", "NI mod 2&3", "NI mod 1") -> (w911:bool[])
            n319 = call "check_ups.vi"() -> ("Error: no voltages read"=w895:bool, "Timestamp last measured"=→"Timestamp last \nmeasured (UPS)":timestamp, "Minimum input voltage measured"=w905:dbl)  [unwired: 8 in, 1 out]
            "Minimum input voltage measured" <- w905
            n320 = property on="Det.P input #" class="DigNum (strict)"() -> ("Value"=w931:i32)  [unwired: 2 in, 2 out]
            n321 = Or Array Elements(Boolean array=w916) -> (logical OR=→"Comm. status":bool)
            n322 = for {
              tunnel: w916 -> [w949] mode=indexing
              tunnel: w911 -> [w948] mode=indexing
              tunnel: [w947] -> w910 mode=indexing
              n323 = And(x=w949, y=w948) -> (x .and. y?=w947:bool)
            }
            n324 = Index Array(array=w932, index=w931) -> (element=w928:dbl)
            n325 = Less?(x=w905, y="UPS Voltage \nLower Threshold") -> (x < y?=w897:bool)
            n326 = Equal?(x=w905, y=-1.0) -> (x = y?=w896:bool)
            n327 = Less?(x=w928, y="Underpressure threshold") -> (x < y?=w926:bool)
            n328 = Build Array(w897, w896, w895) -> (w894:bool[])
            n329 = Or Array Elements(Boolean array=w910) -> (logical OR=w900:bool)
            n330 = Greater?(x=w928, y="Overpressure threshold") -> (0:w927:bool)
            n331 = Or(x=w927, y=w926) -> (x .or. y?=w925:bool)
            "Det. P. warning" <- w925
            n332 = Or Array Elements(Boolean array=w894) -> (logical OR=w893:bool)
            "Warning" <- w893
            n333 = And(x="UPS", y=w893) -> (x .and. y?=w899:bool)
            n334 = And(x=w925, y="Detector Pressure") -> (x .and. y?=w901:bool)
            n335 = Build Array("T 1", "T 2", "T 3", "T 4", "T 5", "T 6") -> (w891:bool[])
            n336 = for {
              tunnel: w890 -> [w950] mode=indexing
              tunnel: w891 -> [w953] mode=indexing
              tunnel: [w952] -> w902 mode=indexing
              tunnel: [w951] -> w917 mode=indexing
              n337 = Less?(x=w950, y="Low Temp threshold") -> (x < y?=w955:bool)
              n338 = Greater?(x=w950, y="High Temp threshold") -> (0:w954:bool)
              n339 = Or(x=w955, y=w954) -> (x .or. y?=w951:bool)
              n340 = And(x=w953, y=w951) -> (x .and. y?=w952:bool)
            }
            n341 = Index Array(array=w917) -> (element #1=→"Boolean":bool, element #2=→"Boolean 2":bool, element #3=→"Boolean 3":bool, element #4=→"Boolean 4":bool, element #5=→"Boolean 5":bool, element #6=→"Boolean 6":bool)  [unwired: 6 in]
            n342 = Build Array (concatenate)(w902, w901, w900, w899) -> (w898:bool[])
            n343 = Or Array Elements(Boolean array=w898) -> (logical OR=w892:bool)
            "Alarm state" <- w892
          }
          frame #8 {
            # "Testing alarm will not interfere"
            # "Act on alarm"
            n344 = Or(x="Test alarm", y=w964) -> (x .or. y?=w965:bool)
            n345 = case shown="True" w965 {
              tunnel: "Test alarm" -> [_ w972]
              tunnel: w962 -> [_ w980]
              tunnel: w958 -> [_ w979]
              tunnel: w961 -> [w968 w970]
              tunnel: "Alarm\nMaster switch" -> [_ w977]
              tunnel: [w968 w971] -> w959
              frame False {
                # "Timer stays at previous value"
              }
              frame True {
                n346 = Get Date/Time In Seconds() -> (seconds since 1Jan1904=w984:timestamp)
                n347 = case shown="True" "\"Sound\" alarm" {
                  frame False {
                  }
                  frame True {
                    n348 = call <vilib>:"Beep.vi"("use system alert? (T)"=FALSE, "duration (msec)"=u32 1000, "frequency (Hz)"="Sound alarm\nFrequency (Hz)") -> ()  [unwired: 9 in]
                  }
                }
                n349 = To Double Precision Float(number=w984) -> (double precision float=w981:dbl)
                n350 = Multiply(x="Repeat Alarm SMS\nevery N minutes", y=60.0) -> (x*y=w973:dbl)
                n351 = Subtract(x=w981, y=w970) -> (x-y=w976:dbl)
                n352 = Greater?(x=w976, y=w973) -> (0:w978:bool)
                n353 = And(x=w977, y=w978) -> (x .and. y?=w975:bool)
                n354 = Or(x=w972, y=w975) -> (x .or. y?=w974:bool)
                n355 = case shown="True" w974 {
                  tunnel: w972 -> [_ w1000]
                  tunnel: w980 -> [_ w1008]
                  tunnel: w979 -> [_ w989]
                  tunnel: [w988 w998] -> w971
                  tunnel: w970 -> [w988 w997]
                  frame False {
                    # "Alarm not armed, or defined time has not yet passed"
                  }
                  frame True {
                    # "Average T in Det."
                    n356 = local read "Det.P input #"() -> (w1013:i32)
                    n357 = case shown="True" w1000 {
                      tunnel: ["Error encountered inXAMS! Status:" "TESTING the XAMS alarm. Status:"] -> w1007
                      tunnel: [w1017 w1020] -> w998
                      tunnel: w997 -> [_ w1020]
                      frame False {
                        n358 = Get Date/Time In Seconds() -> (seconds since 1Jan1904=w1018:timestamp)
                        n359 = To Double Precision Float(number=w1018) -> (double precision float=w1017:dbl)
                      }
                      frame True {
                      }
                    }
                    n360 = for {
                      tunnel: w989 -> [w1022] mode=indexing
                      tunnel: [w1029] -> w992 mode=indexing
                      i -> [w1023]
                      n361 = Format Into String(format string="%.0f", w1023) -> (resulting string=w1027:string)  [unwired: 2 in, 1 out]
                      n362 = Format Into String(format string="%.1f", w1022) -> (resulting string=w1025:string)  [unwired: 2 in, 1 out]
                      n363 = Concatenate Strings("\n" ("format string"), w1027, "     " ("format string"), w1025) -> (w1029:string)
                    }
                    n364 = Index Array(array=w1008, index=w1013) -> (element=w1009:dbl)
                    n365 = Array Size(array=w989) -> (size(s)=w1011:i32)
                    n366 = Add Array Elements(numeric array=w989) -> (sum=w1012:dbl)
                    n367 = Format Into String(format string="%.3f", w1009) -> (resulting string=w1003:string)  [unwired: 2 in, 1 out]
                    n368 = Divide(x=w1012, y=w1011) -> (x/y=w1001:dbl)
                    n369 = Format Date/Time String() -> (date/time string=w1005:string)  [unwired: 3 in]
                    n370 = Format Into String(format string="%.2f", w1001) -> (resulting string=w990:string)  [unwired: 2 in, 1 out]
                    n371 = Concatenate Strings(w1007, "\nDate/time: ", w1005, "\nDetector Pressure: ", w1003, " bar", "\nDetector Temperatures (°C):", "\nCh:   Temp:" ("format string"), w992, "\nAverage detector temperature: ", w990) -> (w996:string)
                    "Alarm (or test) message" <- w996
                    n372 = for {
                      tunnel: w996 -> [w1016]
                      tunnel: "Phone numbers" -> [w1015] mode=indexing
                      n373 = call "send_sms.vi"("Message content"=w1016, "Phone number"=w1015) -> ("standard error"=→"SMS error":string)  [unwired: 8 in, 1 out]
                    }
                  }
                }
              }
            }
            n374 = And(x="Shut off heater \nif Alarm is active", y=w964) -> (x .and. y?=w966:bool)
            "Alarm active 2" <- "Alarm\nMaster switch"
          }
          frame #9 {
            # "Daily e-mail"
            n375 = Get Date/Time In Seconds() -> (seconds since 1Jan1904=w1044:timestamp)
            n376 = To Double Precision Float(number=w1044) -> (double precision float=w1043:dbl)
            n377 = Get Date/Time String(want seconds? (F)=FALSE) -> (time string=w1046:string)  [unwired: 2 in, 1 out]
            n378 = Subtract(x=w1043, y=w1036) -> (x-y=w1042:dbl)
            n379 = Equal?(x=w1046, y="Send status email at time:") -> (x = y?=w1039:bool)
            n380 = Greater?(x=w1042, y=62) -> (0:w1038:bool)
            n381 = Build Array("Send daily email?", w1039, w1038) -> (w1037:bool[])
            n382 = And Array Elements(Boolean array=w1037) -> (logical AND=w1033:bool)
            n383 = Or(x="Send status email now", y=w1033) -> (x .or. y?=w1034:bool)
            n384 = case shown="True" w1034 {
              tunnel: w1031 -> [_ w1051]
              tunnel: w1049 -> [_ w1068]
              tunnel: w1048 -> [_ w1077]
              tunnel: w1036 -> [w1050 _]
              tunnel: [w1050 w1063] -> w1035
              frame False {
              }
              frame True {
                # "Average T in Det."
                n385 = Not Equal To 0?(x="Number of Bonus lines") -> (x != 0?=w1056:bool)
                n386 = case shown="True" w1056 {
                  tunnel: [w1088 w1091] -> w1057
                  tunnel: "Number of Bonus lines" -> [_ w1094]
                  frame False {
                    n387 = Build Array("\n[Flavor text module inactive]") -> (w1088:string[])
                  }
                  frame True {
                    n388 = Build Path(base path=path "C:/Users/xams/Desktop/New XAMS Slow Control", name or relative path="cool_beans.txt") -> (appended path=w1095:path)
                    n389 = call-poly <vilib>:"Read Delimited Spreadsheet.vi"("file path (dialog if empty)"=w1095) -> ("all rows"=w1098:string[][])  [unwired: 9 in, 5 out]
                    n390 = Array Size(array=w1098) -> (size(s)=w1100:i32[])
                    n391 = Index Array(array=w1100) -> (element=w1099:i32)  [unwired: 1 in]
                    n392 = for {
                      N: w1094 -> [_]
                      tunnel: w1099 -> [w1105]
                      tunnel: w1098 -> [w1104]
                      tunnel: [w1101] -> w1092 mode=indexing
                      n393 = Random Number (0-1)() -> (number: 0 to 1=w1108:dbl)
                      n394 = Multiply(x=w1105, y=w1108) -> (x*y=w1107:dbl)
                      n395 = Round To Nearest(number=w1107) -> (nearest integer value=w1106:dbl)
                      n396 = Index Array(array=w1104, index (row)=w1106) -> (element=w1102:string[])  [unwired: 1 in]
                      n397 = Concatenate Strings("\n", w1102) -> (w1101:string)
                    }
                    n398 = Concatenate Strings("\n\nCool beans of the day: ", w1092) -> (w1090:string)
                    n399 = Build Array(w1090) -> (w1091:string[])
                  }
                }
                n400 = local read "Det.P input #"() -> (w1078:i32)
                n401 = for {
                  tunnel: [w1117] -> w1070 mode=indexing
                  tunnel: w1051 -> [w1109] mode=indexing
                  i -> [w1110]
                  n402 = Format Into String(format string="%.0f", w1110) -> (resulting string=w1114:string)  [unwired: 2 in, 1 out]
                  n403 = Format Into String(format string="%.2f", w1109) -> (resulting string=w1112:string)  [unwired: 2 in, 1 out]
                  n404 = Concatenate Strings("\nCh: " ("format string"), w1114, ", Temp: " ("format string"), w1112, "°C." ("format string")) -> (w1117:string)
                }
                n405 = Array Size(array=w1051) -> (size(s)=w1086:i32)
                n406 = Add Array Elements(numeric array=w1051) -> (sum=w1087:dbl)
                n407 = Index Array(array=w1077, index=w1078) -> (element=w1075:dbl)
                n408 = Divide(x=w1087, y=w1086) -> (x/y=w1084:dbl)
                n409 = Format Into String(format string="%.3f", w1075) -> (resulting string=w1073:string)  [unwired: 2 in, 1 out]
                n410 = Format Into String(format string="%.2f", w1084) -> (resulting string=w1067:string)  [unwired: 2 in, 1 out]
                n411 = Select(t="ACTIVE!!!!!", s=w1068, f="inactive.") -> (s? t:f=w1080:string)
                n412 = Concatenate Strings("Hello, XAMS teammembers.", "\n\nThe alarm is currently ", w1080, "\n\nThe latest detector pressure is: ", w1073, " bar." ("format string"), "\nTemperatures inside the detector are:", w1070, "\nThe average detector temperature is ", w1067, "°C." ("format string"), "\n\nThank you for doing your best today, once again!\nRegards, SC.", w1057) -> (w1062:string)
                "Status email preview" <- w1062
                n413 = call "custom_email_program.vi"("mail server"="smtp.nikhef.nl", "return address"="return address", "message"=w1062, "subject ([No Subject])"="XAMS daily status email.", "Email Adresses"="Email Addresses") -> ("error out"=w1054:errorcluster)  [unwired: 6 in]
                n414 = Unbundle By Name(w1054) -> ("code"=→"Email error":i32, "source"=→"source":string)
                n415 = Get Date/Time In Seconds() -> (seconds since 1Jan1904=w1064:timestamp)
                n416 = To Double Precision Float(number=w1064) -> (double precision float=w1063:dbl)
              }
            }
          }
        }
        n417 = Decrement(x="Cycles to execute") -> (x-1=w297:dbl)
        n418 = Decrement(x=w297) -> (x-1=w296:dbl)
        n419 = Greater?(x=w280, y=w296) -> ()  [unwired: 1 out]
        n420 = Decrement(x="Clear data every N cycles") -> (x-1=w277:dbl)
        n421 = Greater?(x=w280, y=w277) -> (0:w279:bool)
        n422 = And(x="Auto-clear data?", y=w279) -> (x .and. y?=w282:bool)
        n423 = Or(x=w282, y="Clear data") -> (x .or. y?=w284:bool)
        n424 = case shown="False" w284 {
          tunnel: w295 -> [w323 _]
          tunnel: [w323 dbl[][] []] -> w294
          tunnel: w293 -> [w322 _]
          tunnel: [w322 w329] -> w292
          tunnel: w291 -> [w321 _]
          tunnel: [w321 w329] -> w290
          tunnel: w289 -> [w320 _]
          tunnel: [w320 w327] -> w288
          tunnel: w287 -> [w319 _]
          tunnel: [w319 w325] -> w286
          tunnel: w280 -> [w318 _]
          tunnel: [w318 0] -> w281
          frame False {
          }
          frame True {
            w329 = 0.0
            n425 = Get Date/Time In Seconds() -> (seconds since 1Jan1904=w326:timestamp)
            n426 = To Double Precision Float(number=w326) -> (double precision float=w328:dbl)
            n427 = Build Array(w326) -> (w325:timestamp[])
            n428 = Build Array(w328, w328) -> (w327:dbl[])
          }
        }
        n429 = Or(x=FALSE, y="stop") -> (x .or. y?=w315:bool)
        "Auto-clear" <- "Auto-clear data?"
      }
    }
    frame True {
    }
  }
  n430 = Array Size(array=w30) -> (size(s)=w33:i32)
  n431 = Decrement(x=w33) -> (x-1=w32:i32)
  n432 = Index Array(array=w30, index #1=w32, index #2=1 ("index")) -> (element #1=w31:timestamp, element #2=w16:timestamp)
  n433 = To Double Precision Float(number=w31) -> (double precision float=w29:dbl)
  n434 = To Double Precision Float(number=w16) -> (double precision float=w28:dbl)
  n435 = flat-sequence {
    tunnel: w23 -> [w1162]
    tunnel: w19 -> [w1134]
    tunnel: w18 -> [w1152]
    tunnel: w11 -> [w1141]
    tunnel: w6 -> [w1138]
    tunnel: w1 -> [w1132]
    frame #0 {
      w1158 = u16 2 items=["1"=1, "2"=2] ("Heater Output (1:1)")
      w1159 = u16 0 items=["Off", "Low (On)", "Medium", "High"] ("Range (0:Off)")
      # "The voltages over the components do NOT get reset by these icons,\nonly the communication gets stopped and references closed."
      # "Important icons! Always press STOP button when done \ninstead of force closing, otherwise these don't get executed"
      # "Turn off heater, shutdown COM"
      # "Error Handling and Post-Processing (EHaPP)"
      n436 = Unbundle(w1162) -> ("VISA resource name out"=w1161:refnum<visa-resource-name>, "error out"=w1160:errorcluster)
      n437 = Unbundle(w1152) -> ("task out"=w1150:refnum<k21>, "error out"=w1148:errorcluster)
      n438 = Unbundle(w1141) -> ("task out"=w1145:refnum<k21>, "error out"=w1143:errorcluster)
      n439 = Unbundle(w1138) -> ("task out"=w1137:refnum<k21>, "error out"=w1136:errorcluster)
      n440 = Index Array(array=w1134) -> (element=w1133:T4)  [unwired: 1 in]
      n441 = Index Array(array=w1132) -> (element #1=w1130:errorcluster, element #2=w1129:errorcluster)  [unwired: 2 in]
      n442 = Merge Errors(w1130, w1129) -> (w1128:errorcluster)
      n443 = Unbundle(w1133) -> ("VISA resource name"=w1153:refnum<visa-resource-name>)  [unwired: 2 out]
      n444 = call <vilib>:"DAQmx Stop Task.vi"("task/channels in"=w1150, "error in"=w1148) -> ("task out"=w1149:refnum<k21>, "error out"=w1147:errorcluster)  [unwired: 12 in]
      n445 = call <vilib>:"DAQmx Stop Task.vi"("task/channels in"=w1145, "error in"=w1143) -> ("task out"=w1144:refnum<k21>, "error out"=w1142:errorcluster)  [unwired: 12 in]
      n446 = call <vilib>:"DAQmx Stop Task.vi"("task/channels in"=w1137, "error in"=w1136) -> ("task out"=w1135:refnum<k21>, "error out"=w1139:errorcluster)  [unwired: 12 in]
      n447 = call <instrlib>:"Configure Output Range and Manual Value.vi"("VISA resource name"=w1161, "Heater Output (1:1)"=w1158, "Range (0:Off)"=w1159, "Manual Output (0.00 %)"=0.0, "error in (no error)"=w1160) -> ("VISA resource name out"=w1156:refnum<visa-resource-name>, "error out"=w1155:errorcluster)  [unwired: 9 in]
      n448 = call <instrlib>:"Close.vi"("VISA resource name"=w1153) -> ("error out"=w1131:errorcluster)  [unwired: 10 in]
      n449 = call <instrlib>:"Close.vi"("error in (no error)"=w1155, "VISA resource name"=w1156) -> ("error out"=w1154:errorcluster)  [unwired: 9 in]
      n450 = call <vilib>:"DAQmx Clear Task.vi"("task in"=w1149, "error in"=w1147) -> ("error out"=w1151:errorcluster)  [unwired: 13 in]
      n451 = call <vilib>:"DAQmx Clear Task.vi"("task in"=w1144, "error in"=w1142) -> ("error out"=w1146:errorcluster)  [unwired: 13 in]
      n452 = call <vilib>:"DAQmx Clear Task.vi"("task in"=w1135, "error in"=w1139) -> ("error out"=w1140:errorcluster)  [unwired: 13 in]
      n453 = Merge Errors(w1131, w1128) -> (w1127:errorcluster)
      n454 = call <vilib>:"Simple Error Handler.vi"("error in (no error)"=w1154) -> ()  [unwired: 4 in, 5 out]
      n455 = call <vilib>:"Simple Error Handler.vi"("error in (no error)"=w1151) -> ()  [unwired: 4 in, 5 out]
      n456 = call <vilib>:"Simple Error Handler.vi"("error in (no error)"=w1146) -> ()  [unwired: 4 in, 5 out]
      n457 = call <vilib>:"Simple Error Handler.vi"("error in (no error)"=w1140) -> ()  [unwired: 4 in, 5 out]
      n458 = call <vilib>:"Simple Error Handler.vi"("error in (no error)"=w1127) -> ()  [unwired: 4 in, 5 out]
    }
  }
  n459 = Subtract(x=w29, y=w28) -> ()  [unwired: 1 out]
  "Started up?" <- w27
